vi "eyecat MAX v2-1_JS_160504.vi"() -> ()   [LabVIEW 2014]
doc: "This VI is an upgrade from the WIN 1_v4 that implements the ageing subrutine"
uses:
  Buttons/String output.ctl
  <vilib>/Utility/miscctls.llb/LVRowAndColumnTypeDef.ctl
  Buttons/Numeric control.ctl
  Buttons/String input.ctl
  Buttons/Numeric indicator.ctl
  Controls Win/Control 3.ctl
  <vilib>/Platform/TimedLoop/XDataNode/nitl_modes.ctl
  <vilib>/Platform/TimedLoop/XDataNode/timing_clust.ctl
  <vilib>/Platform/TimedLoop/XDataNode/wakeup.ctl
  <vilib>/Utility/file.llb/Write To Spreadsheet File (string).vi
  <vilib>/Utility/file.llb/Read From Spreadsheet File (string).vi
  <vilib>/Utility/file.llb/Read From Spreadsheet File (DBL).vi
  <vilib>/regexp/Match Regular Expression.xnode
  <vilib>/Platform/TimedLoop/XDataNode/XDataNode.xnode
  <vilib>/Platform/TimedLoop/XDataNode/XDNodeRunTimeDep.lvlib
panel:
  out "Test Loop":dbl
  out "Mexa_One Emissions":dbl[](array[numeric])
  out "Advanced Logging":bool
  out "Full System":bool
  out "MKS":bool
  in  "Alarm":bool
  in  "Analyser":bool
  in  "MFC":bool
  in  "System":bool
  in  "Ageing":bool
  in  "Performance":bool
  in  "Home":bool
  out "NO":dbl[](array[numeric])
  out "CO":dbl[](array[numeric])
  out "Mexa One":bool
  out "Pressure":dbl
  in  "Duration -1":i32
  in  "Demo Sync":i32
  in  "Demo On":bool
  in  "FlowGuide":bool
  in  "Mean(Off)/Interval(On) 2":bool
  in  "Flow Band %":dbl=1.04
  in  "Flow Sync":i32
  out "Emissions":dbl[](array[numeric])
  in  "Temperature Sync":i32
  in  "TempGuide":bool
  in  "Temp Band %":dbl=1.04
  in  "Mean(Off)/Interval(On)":bool
  in  "MKS 5Hz":bool
  out "output cluster":T2
  out "Lambda":dbl[](array[numeric])
  out "MKS HC":dbl
  in  "HC Index":i32
  out "Open/Closed \nLoop":dbl[](array[numeric])
  out "Air Cyc 2":dbl[](array[numeric])
  in  "Cycle size":i32
  out "ExtAnDn":bool
  out "ExtAnUp":bool
  out "HC Cyc 2":dbl[](array[numeric])
  out "SO Valve 2":dbl[](array[numeric])
  out "SO Valve 1":dbl[](array[numeric])
  out "Air Bal":dbl[](array[numeric])
  out "HC Bal":dbl[](array[numeric])
  out "Air Cyc 1":dbl[](array[numeric])
  out "HC Cyc 1":dbl[](array[numeric])
  out "File name":string
  out "Log?":bool
  out "Connected":bool
  out "Furnace temp 2":dbl
  out "Log interval (seconds)":T1
  in  "Flow rate Age":dbl
  in  "Inlet temp Age":dbl
  out "Stopped?":bool
  in  "Stop Cmd":T1
  out "Connected?":bool
  out "Error":dbl
  out "Iteration Duration":i64
  out "Finished Late? [i-1]":bool
  out "Furnace temp 1":dbl
  out "stop 2":bool
  in  "Enum 1":i16=1
  in  "Acknowledge":bool
  out "Test number":u16
  out "Flag1":bool=TRUE
  out "EditPos Subc":T3
  out "Flag 2":bool=TRUE
  in  "Tab Control":T4(tab)
  out "Warm Up":bool
  in  "Leak Test":bool
  in  "Stop Test":bool
  in  "Log Test Data":bool
  in  "Start Test":bool
  in  "Adv Settings":bool
  out "Doors Unlocked":bool
  in  "Temperature Limit (°C)":T1=1200.0 min=0.0 max=1200.0 step=1.0
  in  "File Name":T5="Test"
  in  "File Path":path=path "C:/DATA LOG"
  out "Fail":bool
  out "Pass":bool
  in  "Select Test Type":T6(radio)
  out "Standby":bool
  out "Doors Open":bool
  out "Extractor Fan On":bool
  out "Test In Progress":bool
  out "Cool Down":bool
  out "System Alarm":bool
  in  "Inlet Temperature (°C)":T1=400.0 min=350.0 max=1000.0 step=1.0
  in  "Inlet LAMBDA Rich":T1=0.9 min=0.85 max=0.96 step=0.001
  in  "Inlet LAMBDA Lean":T1=1.2 min=1.02 max=3.0 step=0.001
  in  "Test Stop temperature (°C)":T1=300.0 min=100.0 max=1000.0 step=1.0
  in  "Test Start Temperature (°C)":T1=125.0 min=0.0 max=500.0 step=1.0
  in  "Furnace Ramp Rate (°C/min)":T1=15.0 min=1.0 max=50.0 step=0.1
  in  "NO:CO Ratio":T1=1.1 min=1.0 max=5.0 step=0.1
  in  "Inlet O2 (%)":T1=0.5 min=0.0 max=14.0 step=0.01
  in  "Inlet LAMBDA":T1=1.0 min=0.6 max=3.0 step=0.001
  out "Space Velocity (h-1)":T7
  out "Vol Flow @ STP (l/min)":T7
  in  "Test Flow Rate(g/s)":T1 min=0.0 max=100.0 step=0.01
  out "Sample Volume (litres)":T7
  in  "Number of Samples":T1=1.0 min=1.0 max=6.0 step=1.0
  in  "Sample Diameter (mm)":T1
  out "CO Theory (%)":T7 format="%#_3g"
  out "CO Theory (%)":T7 format="%#_3g"
  out "HC Theory (%)":T7
  in  "Sample Length (mm)":T1 min=0.0 step=0.5
  in  "NO ppm SW":dbl=500.0 caption="NO (ppm)" min=0.0 max=500.0 step=1.0
  in  "NO ppm Loff":T1 caption="NO ppm"
  in  "Delete sCycle":bool
  in  "Load sCycle":bool
  in  "Save sCycle":bool
  in  "Clear subcycle":bool
  in  "Clear Cycle Pattern":bool
  in  "Save Cycle":bool
  in  "Load Cycle":bool
  in  "Delete Cycle":bool
  out "Test Compiled":bool
  in  "Compile Test Button":bool
  in  "Sub-Cycle List":i32(listbox)=1
  in  "Cycle List":i32(listbox)=2
  out "Total Test Duration (hrs)":T8
  in  "Ageing Gas":enum32{"Radio Selection 1", "Radio Selection 2"}(radio)
  in  "Sub-Cycle Pattern":string[][](table) caption="Subcycle pattern"
  in  "Total Number of Cycles":T1=1.0 min=1.0 max=10000.0 step=1.0
  in  "Cycle Pattern":string[][](table)
  in  "Sub-Cycle Name":T5
  in  "Cycle Name":T5
  out "Heat Exchanger Temperatures (°C)":dynamicdata(graph)
  out "Flow Rate (g/s)":dynamicdata(graph)
  out "Sample Temperatures (°C)":dynamicdata(graph)
  out "System Temperatures (°C)":dynamicdata(graph)
  in  "Graph 1 Box":string(combo)="CO"
  in  "Graph 4 Box":string(combo)="NO"
  in  "Graph 3 Box":string(combo)="Air Cycle 1"
  in  "Graph 2 Box":string(combo)="HC Cycle 1"
  out "MFC Graph 4":dynamicdata(graph)
  out "MFC Graph 3":dynamicdata(graph)
  out "MFC Graph 1":dynamicdata(graph)
  out "MFC Graph 2":dynamicdata(graph)
  out "HC Concentration (ppm)":dynamicdata(graph)
  out "Lambda":dynamicdata(graph)
  out "O2/CO Concentration":dynamicdata(graph)
  out "NO Concentration (ppm)":dynamicdata(graph)
  in  "Purge System":bool
  in  "Alarm ack":bool
  in  "Clear log":bool
  out "Table":string[][](table)
  out "Soft Alarm":bool
  out "Hard Alarm":bool
  # "1% = 0.01"
  # "Test Type"
  # "Test Commands"
  # "System Indicators"
  # "Leak Test"
  # "Catalyst Specification"
  # "Lightoff Settings"
  # "Furnace Lightoff Settings"
  # "Sweep Settings"
  # "CO/HC Lightoff Settings"
  # "0.96 < lambda < 0.85"
  # "1.02< lambda < 1.6"
  # "350 < Tinlet < 1000"
  # "NO Lightoff Settings"
  # "Flow Specification"
  # "Cycle Compiled"
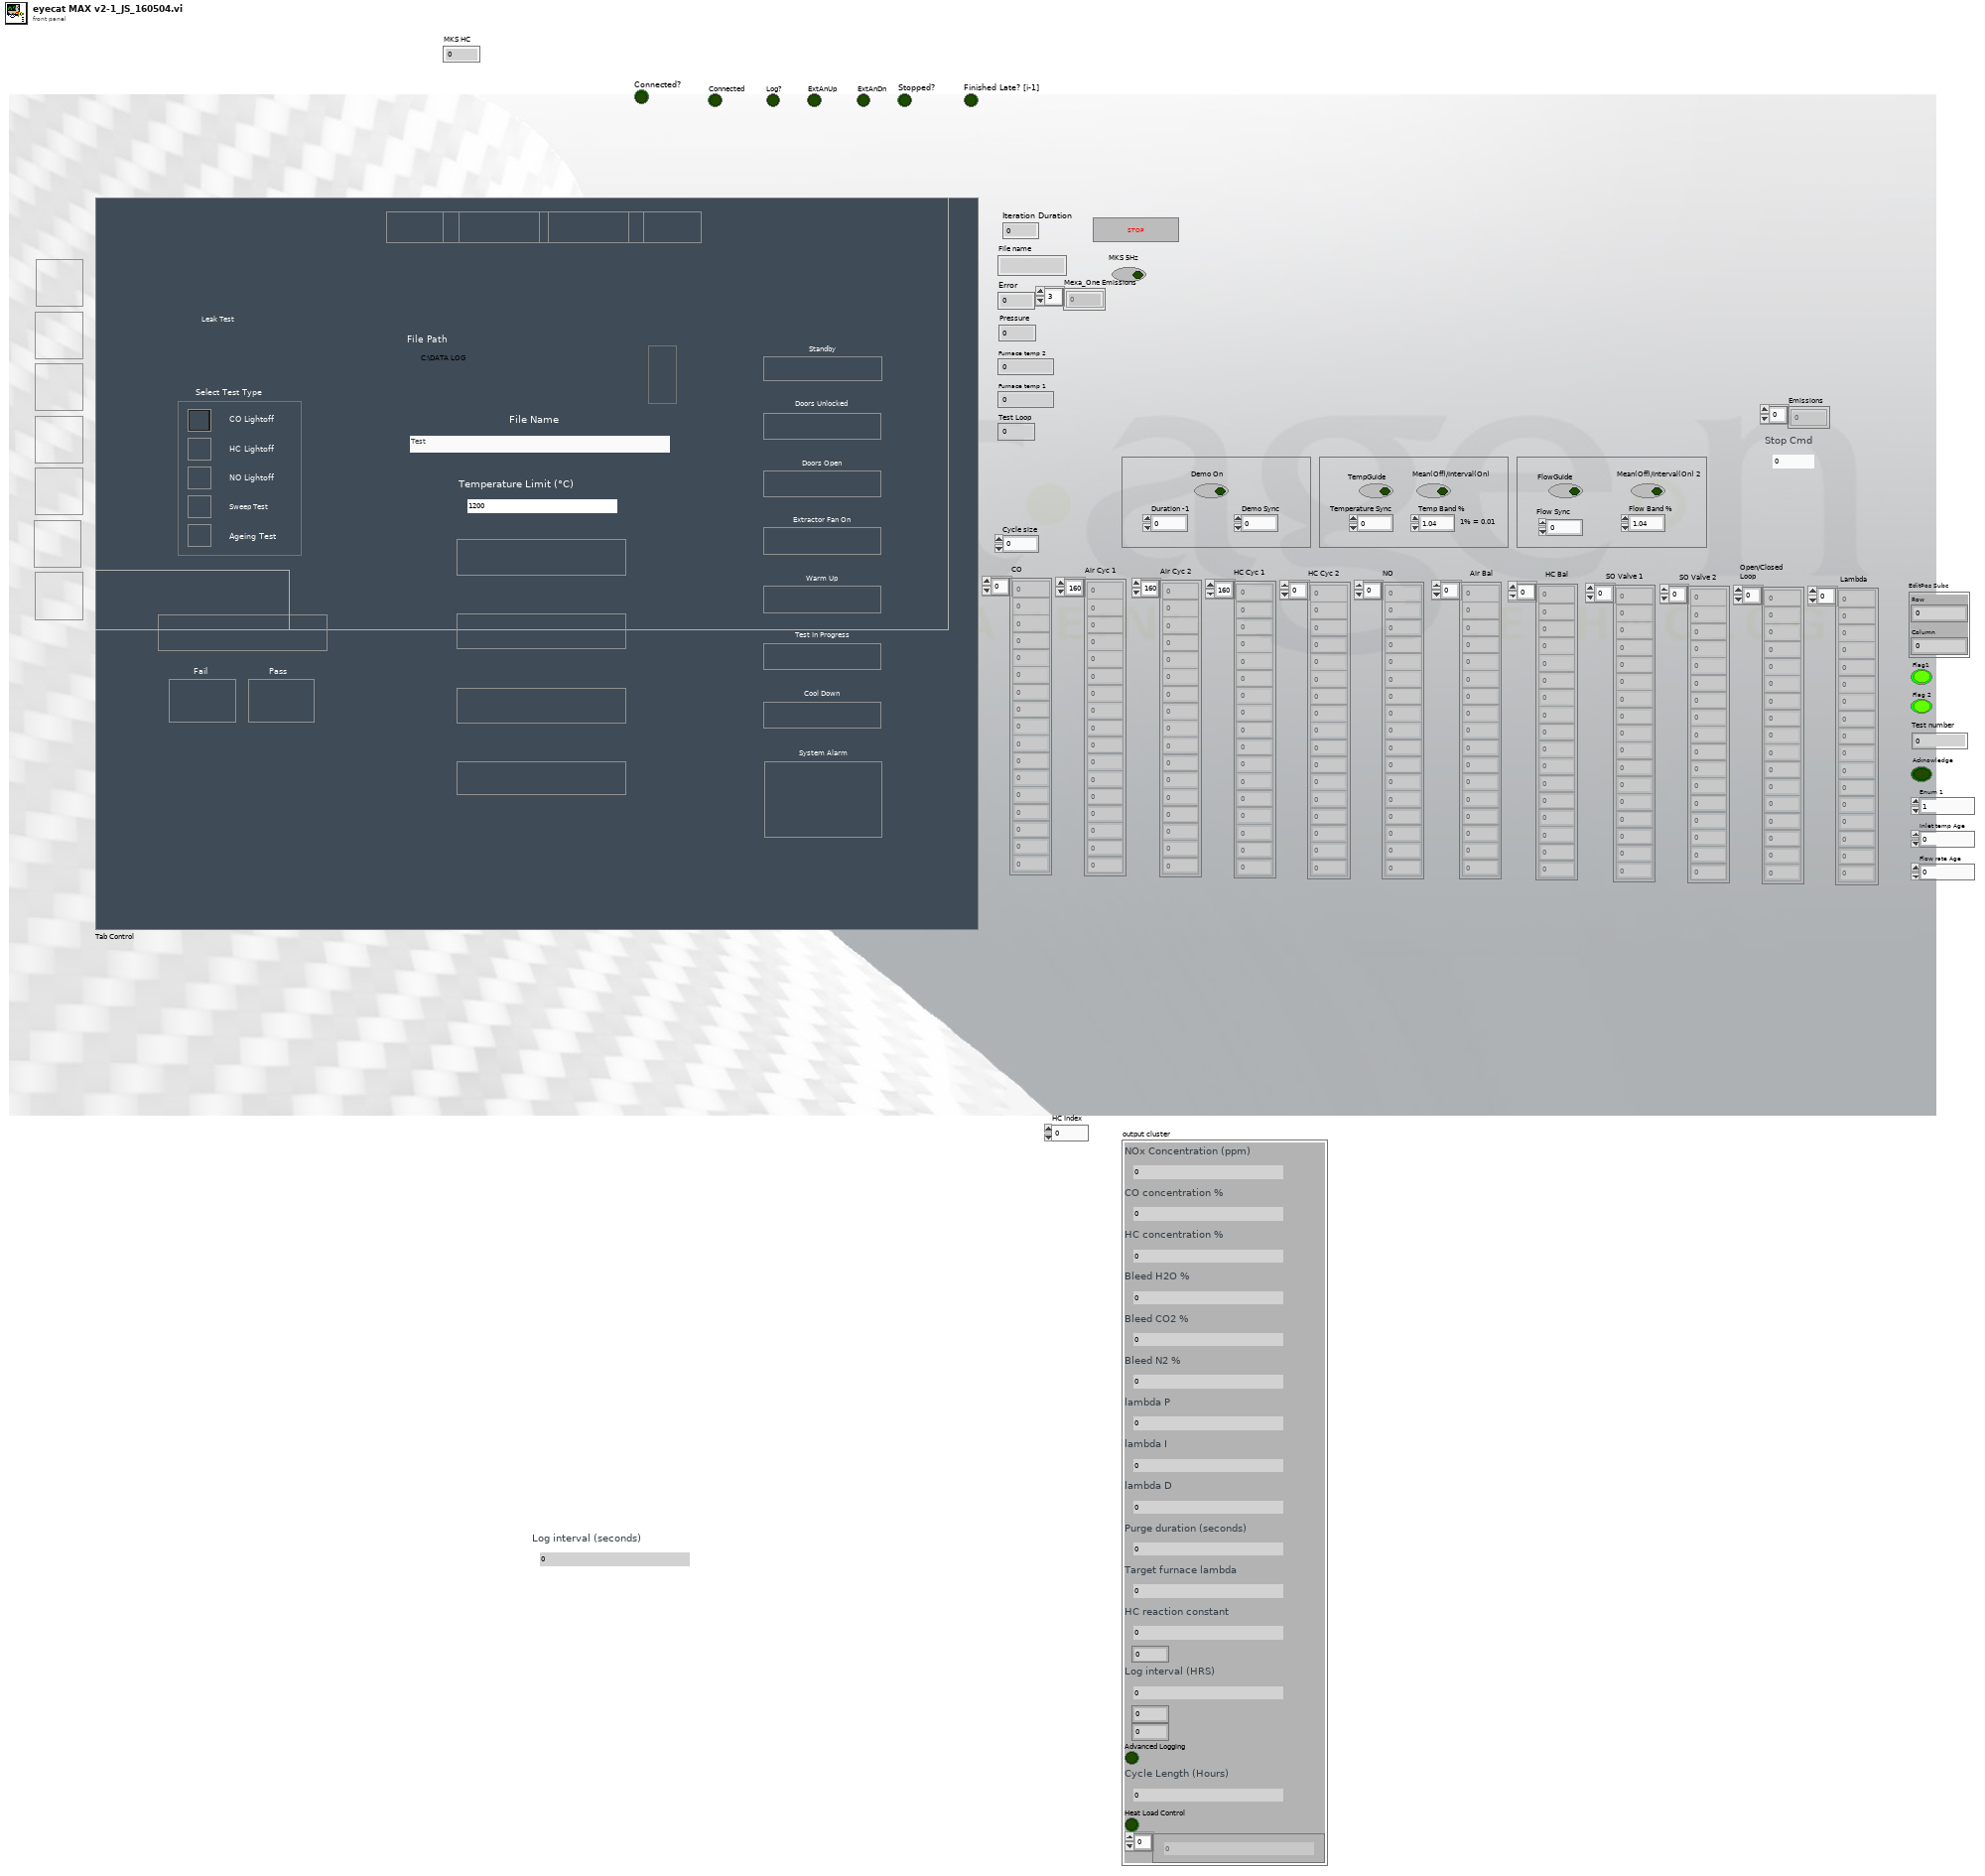
[diagram p1: front panel]
types:
  T1 = typedef "Numeric control.ctl" = dbl
  T2 = cluster{"NOx Concentration (ppm)":T1, "CO concentration %":T1, "HC concentration %":T1, "Bleed H2O %":T1, "Bleed CO2 %":T1, "Bleed N2 %":T1, "lambda P":T1, "lambda I":T1, "lambda D":T1, "Purge duration (seconds)":T1, "Target furnace lambda":T1, "HC reaction constant":T1, i16, "Log interval (HRS)":T1, i16, i16, "Advanced Logging":bool, "Cycle Length (Hours)":T1, "Heat Load Control":bool, T1[]}
  T3 = typedef "LVRowAndColumnTypeDef.ctl" = cluster{"Row":i32, "Column":i32}
  T4 = enum32{"MAIN", "PERFORMANCE TEST SETUP", "AGEING TEST SETUP", "SYSTEM DATA", "MFC", "ANALYSER DATA", "ALARM LOG"}
  T5 = typedef "String input.ctl" = string
  T6 = enum32{"CO Lightoff", "HC Lightoff", "NO Lightoff", "Sweep Test", "Ageing Test"}
  T7 = typedef "Numeric indicator.ctl" = dbl
  T8 = typedef "String output.ctl" = string
  T9 = typedef "XDNodeRunTimeDep.lvlib/nitl_modes.ctl" = enum32{"No Change", "Process missed periods, maintain original phase", "Discard missed periods, maintain original phase", "Process missed periods, ignore original phase", "Discard missed periods, ignore original phase"}
  T10 = typedef "Control 3.ctl" = enum16{"main", "start test", "save subc", "load subc", "delete subc", "clear table 1", "update list 1", "save cycle", "load cycle", "delete cycle", "clear table 2", "update list 2", "calc HC CO", "Total time calc", "update Cycle pattern ", "load cycle name", "convert to num", "load test array", "check scycle name", "check cycle name", "Multigas connect", "Multigas disconnect", "Leak Test"}
  T11 = enum8{"Enabled", "Disabled", "Disabled and Grayed Out"}
  T12 = typedef "XDNodeRunTimeDep.lvlib/timing_clust.ctl" = cluster{"Expected End [f-1]":u64, "Actual End [f-1]":u64, "Finished Late? [f-1]":bool, "Expected End [i-1]":u64, "Actual End [i-1]":u64, "Finished Late? [i-1]":bool, "Expected Start [i]":u64, "Actual Start [i]":u64, "Expected Start [f]":u64, "Actual Start [f]":u64, "Source Name":string, "Structure Name":string, "Period":i64, "Deadline":i64, "Offset":i64, "Start":i64, "Priority":i32, "Timeout":i32, "Mode":T9, "Wakeup Reason":T13, "Error":errorcluster, "Source Type":string, "Secondary Source Type":string, "Global End Time":u64, "Global Start Time":u64, "Frame Duration":u64, "Iteration Duration":u64, "Assigned CPU":i32, "I/O Scan Engine Mode":u32}
  T13 = typedef "XDNodeRunTimeDep.lvlib/wakeup.ctl" = enum32{"Normal", "Aborted", "Asynchronous wakeup", "Timing source error", "Timed loop error", "Timeout"}
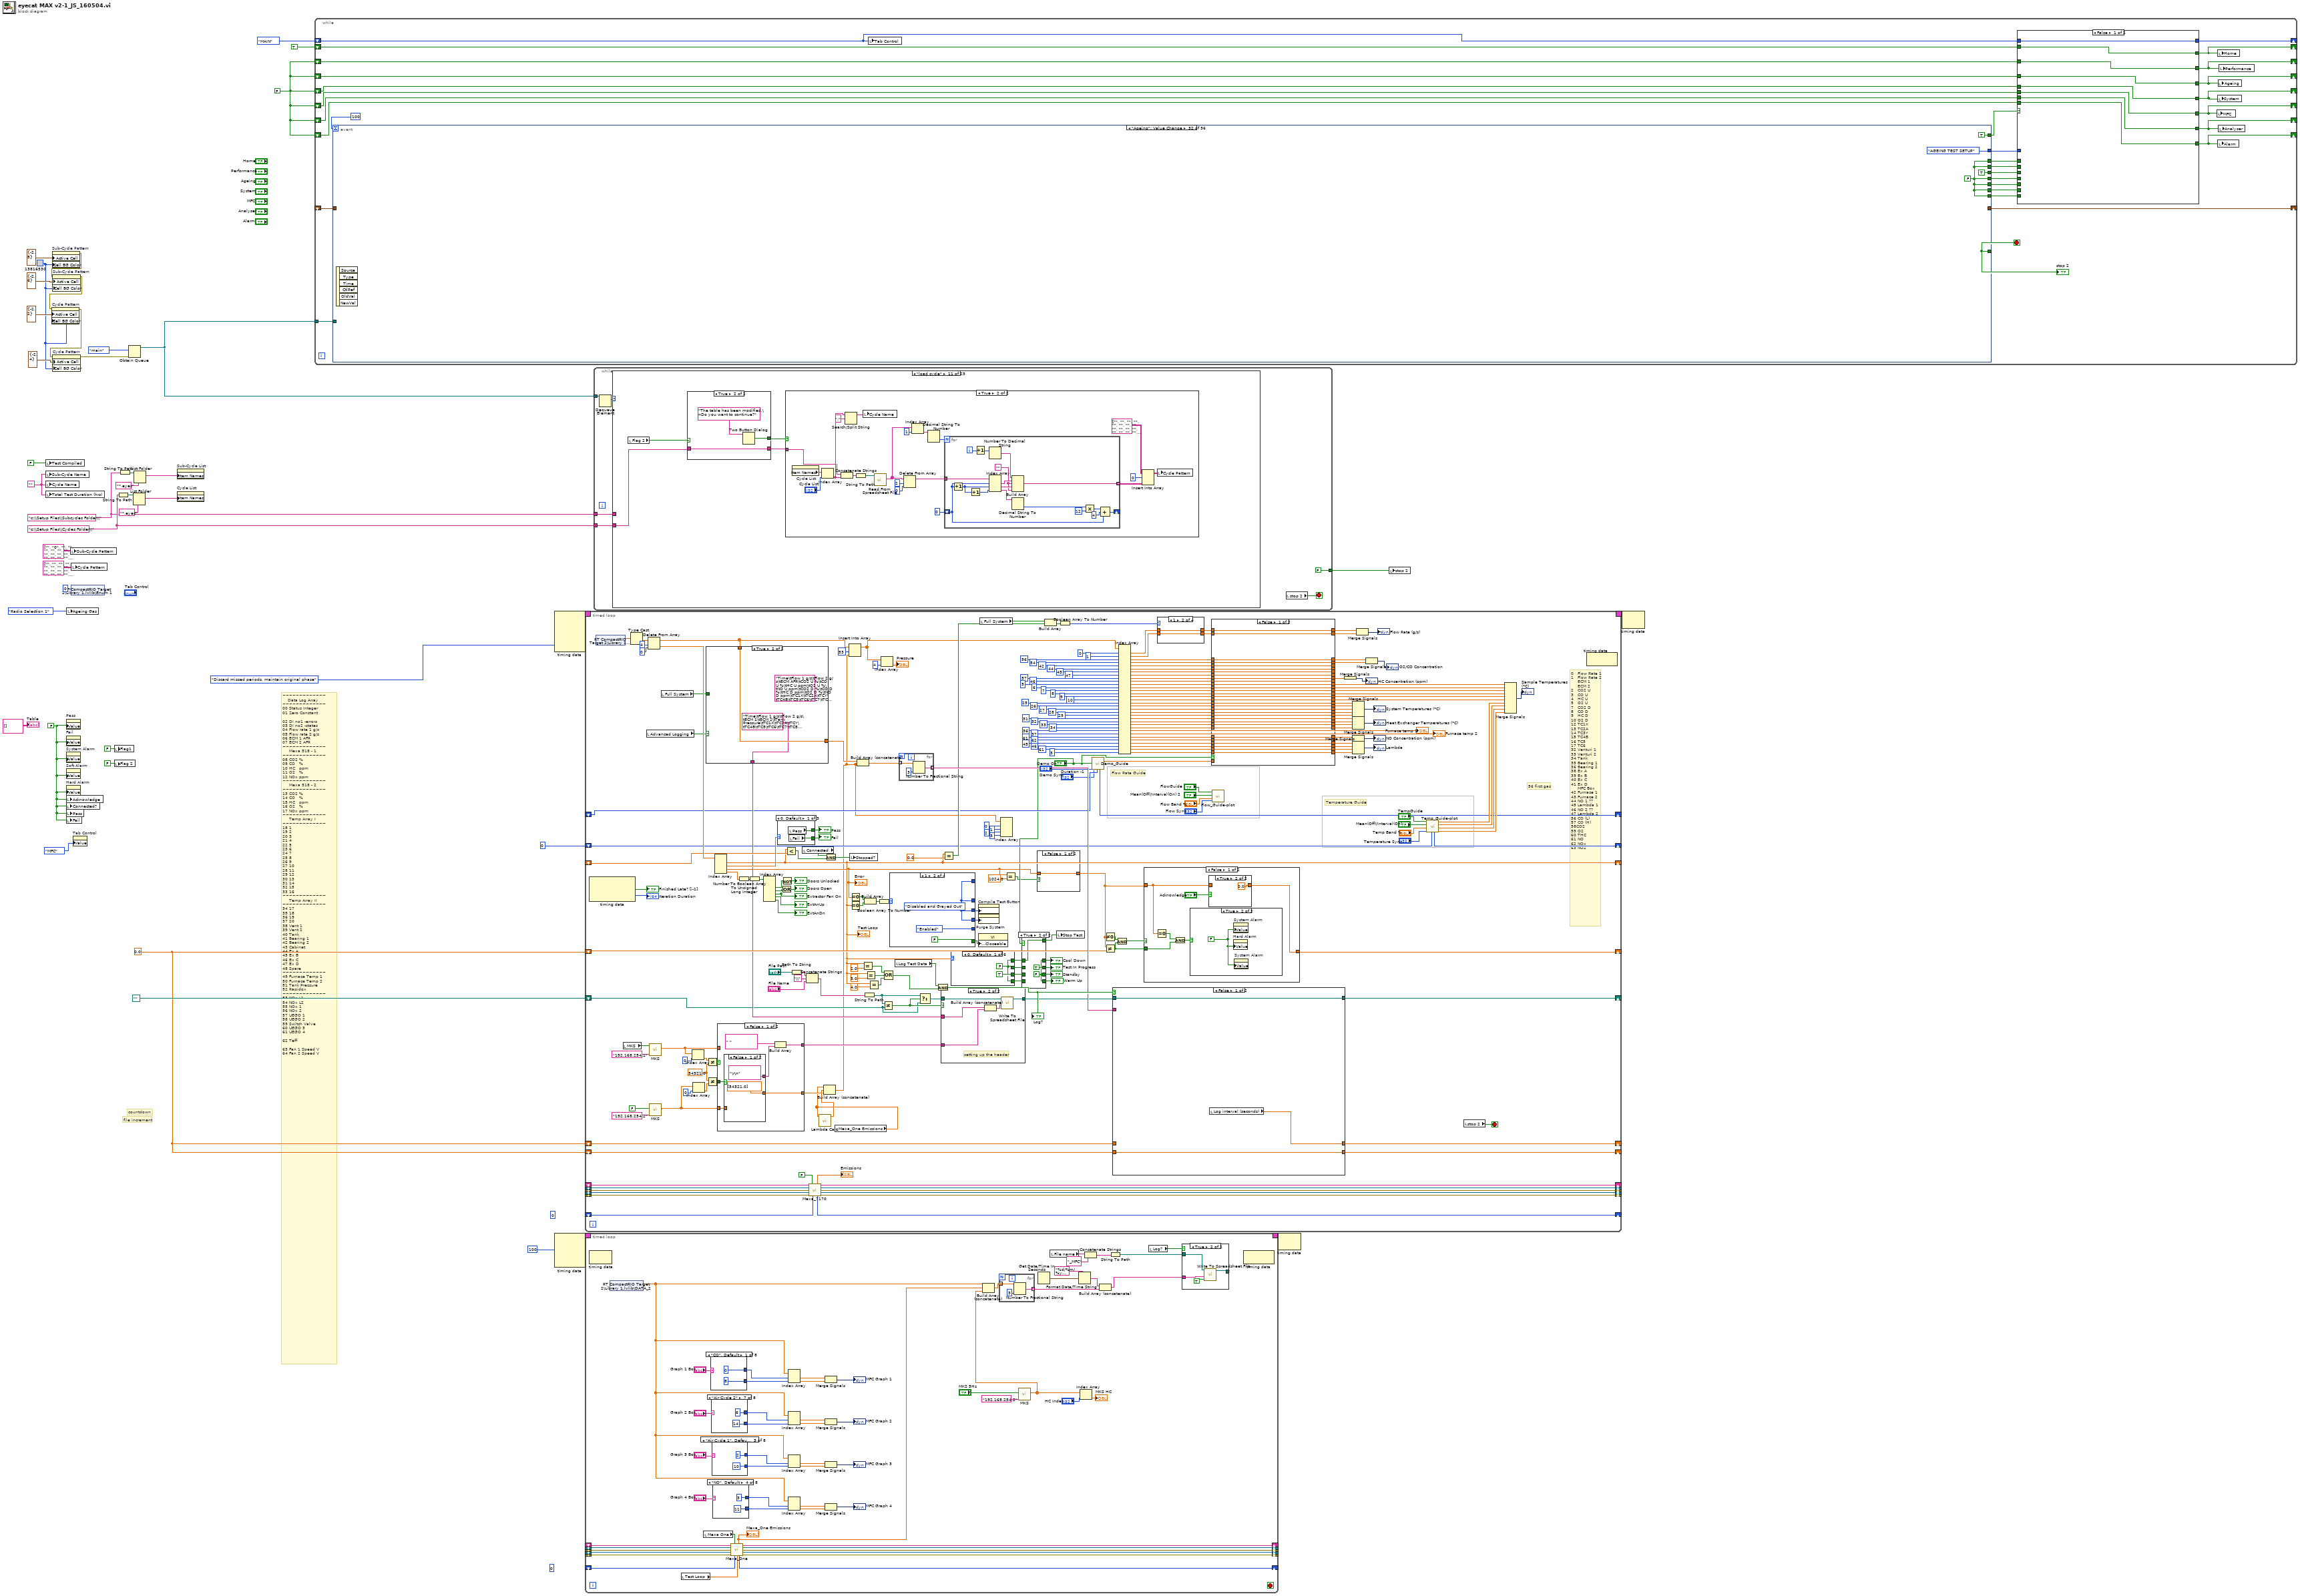
[diagram p0: block diagram]
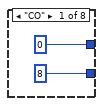
[diagram p2: hidden frame]
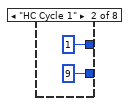
[diagram p3: hidden frame]
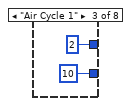
[diagram p4: hidden frame]
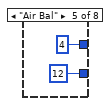
[diagram p5: hidden frame]
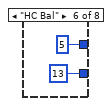
[diagram p6: hidden frame]
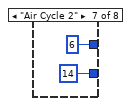
[diagram p7: hidden frame]
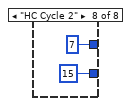
[diagram p8: hidden frame]
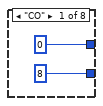
[diagram p9: hidden frame]
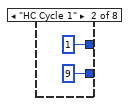
[diagram p10: hidden frame]
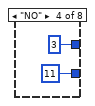
[diagram p11: hidden frame]
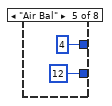
[diagram p12: hidden frame]
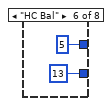
[diagram p13: hidden frame]
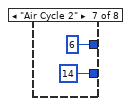
[diagram p14: hidden frame]
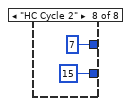
[diagram p15: hidden frame]
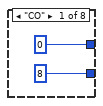
[diagram p16: hidden frame]
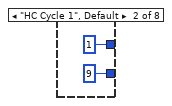
[diagram p17: hidden frame]
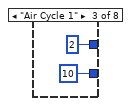
[diagram p18: hidden frame]
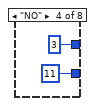
[diagram p19: hidden frame]
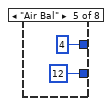
[diagram p20: hidden frame]
diagram:
  (unwired) 0 ("index")
  w2 = FALSE
  (unwired) 0 ("index")
  w10 = FALSE
  w9 = 0.0 ("y")
  w25 = ""
  w28 = "c:\\Setup Files\\Cycles Folder\\"
  w34 = u32 13816530
  w26 = "c:\\Setup Files\\Subcycles Folder\\"
  # "~~~~~~~~~~~~~\n    Data Log Array\n~~~~~~~~~~~~~\n00 Status Integer\n01 Zero Constant\n\n02 DI no1 -errors\n03 DI no2 -states\n04 Flow rate 1 g/s\n05 Flow rate 2 g/s\n06 ECM 1 AFR\n07 ECM 2 AFR\n~~~~~~~~~~~~~\n     Mexa 518 - 1\n~~~~~~~~~~~~~\n08 CO2 %\n09 CO   %\n10 HC   ppm\n11 O2   %\n12 NOx ppm\n~~~~~~~~~~~~~\n     Mexa 518 - 2\n~~~~~~~~~~~~~\n13 CO2 %\n14 CO   %\n15 HC   ppm\n16 O2   %\n17 NOx ppm\n~~~~~~~~~~~~~\n     Temp Array I\n~~~~~~~~~~~~~\n18 1\n19 2 \n20 3\n21 4\n22 5\n23 6\n24 7\n25 8\n26 9\n27 10\n28 11\n29 12\n30 13\n31 14\n32 15\n33 16\n~~~~~~~~~~~~~\n     Temp Array II\n~~~~~~~~~~~~~\n34 17\n35 18\n36 19\n37 20\n38 Vent 1\n39 Vent 2\n40 Tank\n41 Bearing 1\n42 Bearing 2\n43 Cabinet\n44 Ex A\n45 Ex B\n46 Ex C\n47 Ex D\n48 Spare\n~~~~~~~~~~~~~\n49 Furnace Temp 1\n50 Furnace Temp 2\n51 Tank Pressure\n52 Rapidox\n~~~~~~~~~~~~~\n53 NOx L1\n54 NOx L2\n55 NOx 1\n56 NOx 2\n57 UEGO 1\n58 UEGO 2\n59 Switch Valve\n60 UEGO 3\n61 UEGO 4\n\n62 Teff\n\n63 Fan 1 Speed V\n64 Fan 2 Speed V"
  # "file increment"
  # "countdown"
  n1 = local write "Test Compiled"(FALSE ("Cycle Compiled")) -> ()
  n2 = local write "Sub-Cycle Name"(w25) -> ()
  n3 = local write "Cycle Name"(w25) -> ()
  n4 = local write "Total Test Duration (hrs)"(w25) -> ()
  n5 = property on="Sub-Cycle Pattern" class="Tbl (strict)"("Active Cell"=T3 {"Row"=-2, "Column"=5} ("Active Cell:Active Cell"), "Cell BG Color"=w34) -> (error out=w39:errorcluster)  [unwired: 2 in, 1 out]
  n6 = property on="Sub-Cycle Pattern" class="Tbl (strict)"(error in=w39, "Active Cell"=T3 {"Row"=-2, "Column"=6} ("Active Cell:Active Cell"), "Cell BG Color"=w34) -> (error out=w38:errorcluster)  [unwired: 1 in, 1 out]
  n7 = property on="Cycle Pattern" class="Tbl (strict)"(error in=w38, "Active Cell"=T3 {"Row"=-2, "Column"=2} ("Active Cell:Active Cell"), "Cell BG Color"=w34) -> (error out=w36:errorcluster)  [unwired: 1 in, 1 out]
  n8 = property on="Cycle Pattern" class="Tbl (strict)"(error in=w36, "Active Cell"=T3 {"Row"=-2, "Column"=4} ("Active Cell:Active Cell"), "Cell BG Color"=w34) -> (error out=w33:errorcluster)  [unwired: 1 in, 1 out]
  n9 = property on="Pass" class="Bool (strict)"("Value"=w10) -> ()  [unwired: 2 in, 2 out]
  n10 = property on="Fail" class="Bool (strict)"("Value"=w10) -> ()  [unwired: 2 in, 2 out]
  n11 = property on="System Alarm" class="Bool (strict)"("Value"=w10) -> ()  [unwired: 2 in, 2 out]
  n12 = property on="Soft Alarm" class="Bool (strict)"("Value"=w10) -> ()  [unwired: 2 in, 2 out]
  n13 = property on="Hard Alarm" class="Bool (strict)"("Value"=w10) -> ()  [unwired: 2 in, 2 out]
  n14 = local write "Acknowledge"(w10) -> ()
  n15 = local write "Connected?"(w10) -> ()
  n16 = local write "Pass"(w10) -> ()
  n17 = local write "Fail"(w10) -> ()
  n18 = local write "Ageing Gas"(enum32{"Radio Selection 1", "Radio Selection 2"}."Radio Selection 1" ("Ageing Gas")) -> ()
  n19 = local write "Sub-Cycle Pattern"(string[][] [["", "0", "", "", "", "", "", "", "", "", "", "", ""], ["", "", "", "", "", "", "", "", "", "", "", "", ""], ["", "", "", "", "", "", "", "", "", "", "", "", ""], ["", "", "", "", "", "", "", "", "", "", "", "", ""], ["", "", "", "", "", "", "", "", "", "", "", "", ""], ["", "", "", "", "", "", "", "", "", "", "", "", ""], ["", "", "", "", "", "", "", "", "", "", "", "", ""], ["", "", "", "", "", "", "", "", "", "", "", "", ""], ["", "", "", "", "", "", "", "", "", "", "", "", ""], ["", "", "", "", "", "", "", "", "", "", "", "", ""], ["", "", "", "", "", "", "", "", "", "", "", "", ""], ["", "", "", "", "", "", "", "", "", "", "", "", ""], ["", "", "", "", "", "", "", "", "", "", "", "", ""], ["", "", "", "", "", "", "", "", "", "", "", "", ""], ["", "", "", "", "", "", "", "", "", "", "", "", ""], ["", "", "", "", "", "", "", "", "", "", "", "", ""], ["", "", "", "", "", "", "", "", "", "", "", "", ""], ["", "", "", "", "", "", "", "", "", "", "", "", ""], ["", "", "", "", "", "", "", "", "", "", "", "", ""], ["", "", "", "", "", "", "", "", "", "", "", "", ""], ["", "", "", "", "", "", "", "", "", "", "", "", ""], ["", "", "", "", "", "", "", "", "", "", "", "", ""], ["", "", "", "", "", "", "", "", "", "", "", "", ""], ["", "", "", "", "", "", "", "", "", "", "", "", ""], ["", "", "", "", "", "", "", "", "", "", "", "", ""], ["", "", "", "", "", "", "", "", "", "", "", "", ""], ["", "", "", "", "", "", "", "", "", "", "", "", ""], ["", "", "", "", "", "", "", "", "", "", "", "", ""], ["", "", "", "", "", "", "", "", "", "", "", "", ""], ["", "", "", "", "", "", "", "", "", "", "", "", ""], ["", "", "", "", "", "", "", "", "", "", "", "", ""]]) -> ()
  n20 = local write "Cycle Pattern"(string[][] [["", "", "", "", ""], ["", "", "", "", ""], ["", "", "", "", ""], ["", "", "", "", ""], ["", "", "", "", ""], ["", "", "", "", ""], ["", "", "", "", ""], ["", "", "", "", ""], ["", "", "", "", ""], ["", "", "", "", ""], ["", "", "", "", ""], ["", "", "", "", ""], ["", "", "", "", ""], ["", "", "", "", ""], ["", "", "", "", ""], ["", "", "", "", ""], ["", "", "", "", ""], ["", "", "", "", ""], ["", "", "", "", ""], ["", "", "", "", ""], ["", "", "", "", ""], ["", "", "", "", ""], ["", "", "", "", ""], ["", "", "", "", ""], ["", "", "", "", ""], ["", "", "", "", ""], ["", "", "", "", ""], ["", "", "", "", ""], ["", "", "", "", ""], ["", "", "", "", ""], ["", "", "", "", ""]]) -> ()
  n21 = shared-variable "RT CompactRIO Target 2\\Library 1.lvlib\\Enum 1"(u16 0 ("Enum 1")) -> ()  [unwired: 1 in, 1 out]
  n22 = property on="Tab Control" class="TabCtl (strict)"("Value"=T4."MFC" ("Tab Control")) -> ()  [unwired: 2 in, 2 out]
  n23 = local write "Flag1"(FALSE) -> ()
  n24 = local write "Flag 2"(FALSE) -> ()
  n25 = String To Path(string=w28) -> (path=w29:path)
  n26 = String To Path(string=w26) -> (path=w31:path)
  n27 = Obtain Queue(element data type=Control_3."main" ("Enum"), error in (no error)=w33) -> (queue out=w42:refnum<queue>)  [unwired: 3 in, 2 out]
  n28 = List Folder(path=w29, pattern="*.eyec") -> (filenames=w30:string[])  [unwired: 2 in, 3 out]
  n29 = List Folder(path=w31, pattern="*.eyes") -> (filenames=w32:string[])  [unwired: 2 in, 3 out]
  n30 = property on="Sub-Cycle List" class="LstBox (strict)"("Item Names"=w32) -> ()  [unwired: 2 in, 2 out]
  n31 = property on="Cycle List" class="LstBox (strict)"("Item Names"=w30) -> ()  [unwired: 2 in, 2 out]
  n32 = while {
    tunnel: w42 -> [w73]
    shift-right: [w71] -> _
    shift-left: _ -> [w70]
    shift-right: [w68] -> _
    shift-left: T4."MAIN" ("Tab Control") -> [w67]
    shift-right: [w56] -> _
    shift-left: w2 -> [w49]
    shift-right: [w57] -> _
    shift-left: TRUE -> [w50]
    shift-right: [w55] -> _
    shift-left: w2 -> [w44]
    shift-right: [w54] -> _
    shift-left: w2 -> [w45]
    shift-right: [w53] -> _
    shift-left: w2 -> [w46]
    shift-right: [w52] -> _
    shift-left: w2 -> [w47]
    shift-right: [w51] -> _
    shift-left: w2 -> [w48]
    stop <- w69 stop-if-true
    n33 = event shown="[31] \"Ageing\": Value Change" {
      selector: _ -> [_ _ _ _ _ _ _ _ _ _ _ _ _ _ _ _ _ _ _ _ _ _ _ _ _ _ _ _ _ _ _ _ _ _ _ _]
      dyn-events: _ -> [_ _ _ _ _ _ _ _ _ _ _ _ _ _ _ _ _ _ _ _ _ _ _ _ _ _ _ _ _ _ _ _ _ _ _ _]
      timeout: 100 -> [_ _ _ _ _ _ _ _ _ _ _ _ _ _ _ _ _ _ _ _ _ _ _ _ _ _ _ _ _ _ _ _ _ _ _ _]
      tunnel: w73 -> [w92 w94 _ w103 w111 w118 w125 w136 w140 w151 w156 w159 w164 w186 w194 w195 _ _ _ _ w239 w250 _ w342 w366 _ w380 _ _ _ _ _ _ _ _ _]
      tunnel: [w90 w93 _ w104 w110 w117 w124 w135 w138 w146 w153 w158 w162 w183 _ _ _ _ _ _ _ _ _ _ _ _ _ _ _ _ _ _ _ _ _ _] -> w71
      tunnel: w70 -> [w90 w93 _ w104 w110 w117 w123 w135 w138 w146 w153 w158 w162 w183 _ _ _ _ _ _ _ _ _ _ _ _ _ _ _ _ _ _ _ _ _ _]
      tunnel: [_ _ w96 _ _ _ _ _ _ _ _ _ _ _ _ _ _ _ _ _ _ _ _ _ _ _ _ _ _ _ _ _ _ _ _ _] -> w69
      tunnel: [_ _ _ _ _ _ _ _ _ _ _ _ _ _ _ _ _ _ _ _ _ _ _ _ _ _ _ _ _ TRUE TRUE TRUE TRUE TRUE TRUE TRUE] -> w66
      tunnel: [_ _ _ _ _ _ _ _ _ _ _ _ _ _ _ _ _ _ _ _ _ _ _ _ _ _ _ _ _ T4."MAIN" ("Tab Control") T4."PERFORMANCE TEST SETUP" ("Tab Control") T4."AGEING TEST SETUP" ("Tab Control") T4."SYSTEM DATA" ("Tab Control") T4."MFC" ("Tab Control") T4."ANALYSER DATA" ("Tab Control") T4."ALARM LOG" ("Tab Control")] -> w65
      tunnel: [_ _ _ _ _ _ _ _ _ _ _ _ _ _ _ _ _ _ _ _ _ _ _ _ _ _ _ _ _ TRUE w391 w395 w399 w403 w408 w411] -> w64
      tunnel: [_ _ _ _ _ _ _ _ _ _ _ _ _ _ _ _ _ _ _ _ _ _ _ _ _ _ _ _ _ w388 TRUE w395 w399 w403 w408 w411] -> w63
      tunnel: [_ _ _ _ _ _ _ _ _ _ _ _ _ _ _ _ _ _ _ _ _ _ _ _ _ _ _ _ _ w388 w391 TRUE w399 w403 w408 w411] -> w62
      tunnel: [_ _ _ _ _ _ _ _ _ _ _ _ _ _ _ _ _ _ _ _ _ _ _ _ _ _ _ _ _ w388 w391 w395 TRUE w403 w408 w411] -> w61
      tunnel: [_ _ _ _ _ _ _ _ _ _ _ _ _ _ _ _ _ _ _ _ _ _ _ _ _ _ _ _ _ w388 w391 w395 w399 TRUE w408 w411] -> w60
      tunnel: [_ _ _ _ _ _ _ _ _ _ _ _ _ _ _ _ _ _ _ _ _ _ _ _ _ _ _ _ _ w388 w391 w395 w399 w403 TRUE w411] -> w59
      tunnel: [_ _ _ _ _ _ _ _ _ _ _ _ _ _ _ _ _ _ _ _ _ _ _ _ _ _ _ _ _ w388 w391 w395 w399 w403 w408 TRUE] -> w58
      event Timeout {
        n34 = event-data() -> ()  [unwired: 1 in, 2 out]
        n35 = Enqueue Element(queue=w92, element=Control_3."main" ("Enum")) -> ()  [unwired: 2 in, 3 out]
      }
      event "Clear subcycle": Value Change {
        n36 = event-data() -> ()  [unwired: 1 in, 5 out]
        n37 = Enqueue Element(queue=w94, element=Control_3."clear table 1" ("Enum")) -> ()  [unwired: 2 in, 3 out]
      }
      event Panel Close? {
        n38 = event-data() -> ()  [unwired: 1 in, 3 out]
        n39 = Two Button Dialog(message="This command will close Eyecat!\nDo you wish to continue?", 1:"No" ("F button name (\"Cancel\")"), 2:"Yes" ("T button name (\"OK\")")) -> (T button?=w96:bool)
        n40 = Not(x=w96) -> (.not. x?=w97:bool)
        n41 = event-data("Discard?"=w97) -> ()  [unwired: 1 in, 1 out]
      }
      event "Save sCycle": Value Change {
        n42 = event-data() -> ()  [unwired: 1 in, 5 out]
        n43 = local read "Sub-Cycle Pattern"() -> (w101:string[][])
        n44 = call "Time column check.vi"("Array"=w101) -> ("Mistake?"=w102:bool)  [unwired: 10 in]
        n45 = case shown="False" w102 {
          tunnel: w103 -> [w105 _]
          frame False {
            n46 = Enqueue Element(queue=w105, element=Control_3."save subc") -> (queue out=w107:refnum<queue>)  [unwired: 2 in, 2 out]
            n47 = Enqueue Element(queue=w107, element=Control_3."update list 1") -> ()  [unwired: 2 in, 3 out]
          }
          frame True {
            n48 = One Button Dialog(message="The time sequence is incorrect!\nReview and save again!") -> ()  [unwired: 1 in, 1 out]
          }
        }
      }
      event "Load sCycle": Value Change {
        n49 = event-data() -> ()  [unwired: 1 in, 5 out]
        n50 = Enqueue Element(queue=w111, element=Control_3."load subc") -> ()  [unwired: 2 in, 3 out]
      }
      event "Delete sCycle": Value Change {
        n51 = event-data() -> ()  [unwired: 1 in, 5 out]
        n52 = Enqueue Element(queue=w118, element=Control_3."delete subc") -> (queue out=w120:refnum<queue>)  [unwired: 2 in, 2 out]
        n53 = Enqueue Element(queue=w120, element=Control_3."update list 1") -> (queue out=w116:refnum<queue>)  [unwired: 2 in, 2 out]
        n54 = Enqueue Element(queue=w116, element=Control_3."update Cycle pattern ") -> (queue out=w113:refnum<queue>)  [unwired: 2 in, 2 out]
        n55 = Enqueue Element(queue=w113, element=Control_3."Total time calc") -> ()  [unwired: 2 in, 3 out]
      }
      event "Sub-Cycle Pattern": Mouse Down; "Sub-Cycle Pattern": Value Change {
        n56 = event-data() -> ()  [unwired: 1 in, 3 out]
        n57 = property on="Sub-Cycle Pattern" class="Tbl (strict)"() -> ("EditPos"=w124:T3)  [unwired: 2 in, 2 out]
        n58 = Unbundle By Name(w124) -> ("Row"=w126:i32)  [unwired: 1 out]
        n59 = Less?(x=w126, y=30) -> (x < y?=w128:bool)
        n60 = case shown="True" w128 {
          tunnel: w125 -> [_ w133]
          frame False {
            n61 = One Button Dialog(message="This table is limited to 30 entries!") -> ()  [unwired: 1 in, 1 out]
          }
          frame True {
            n62 = Enqueue Element(queue=w133, element=Control_3."convert to num") -> (queue out=w132:refnum<queue>)  [unwired: 2 in, 2 out]
            n63 = Enqueue Element(queue=w132, element=Control_3."calc HC CO") -> ()  [unwired: 2 in, 3 out]
          }
        }
        "EditPos Subc" <- w123
        "Flag1" <- TRUE
      }
      event "Clear Cycle Pattern": Value Change {
        n64 = event-data() -> ()  [unwired: 1 in, 5 out]
        n65 = Enqueue Element(queue=w136, element=Control_3."clear table 2" ("Enum")) -> ()  [unwired: 2 in, 3 out]
        n66 = local write "Test Compiled"(FALSE ("Test Compiled")) -> ()
      }
      event "Save Cycle": Value Change {
        n67 = event-data() -> ()  [unwired: 1 in, 5 out]
        n68 = Enqueue Element(queue=w140, element=Control_3."update Cycle pattern ") -> (queue out=w139:refnum<queue>)  [unwired: 2 in, 2 out]
        n69 = Enqueue Element(queue=w139, element=Control_3."save cycle") -> (queue out=w143:refnum<queue>)  [unwired: 2 in, 2 out]
        n70 = Enqueue Element(queue=w143, element=Control_3."update list 2") -> ()  [unwired: 2 in, 3 out]
      }
      event "Load Cycle": Value Change {
        n71 = event-data() -> ()  [unwired: 1 in, 5 out]
        n72 = Enqueue Element(queue=w151, element=Control_3."load cycle") -> (queue out=w149:refnum<queue>)  [unwired: 2 in, 2 out]
        n73 = Enqueue Element(queue=w149, element=Control_3."update Cycle pattern ") -> (queue out=w148:refnum<queue>)  [unwired: 2 in, 2 out]
        n74 = local write "Test Compiled"(FALSE ("Test Compiled")) -> ()
        n75 = Enqueue Element(queue=w148, element=Control_3."Total time calc") -> ()  [unwired: 2 in, 3 out]
      }
      event "Delete Cycle": Value Change {
        n76 = event-data() -> ()  [unwired: 1 in, 5 out]
        n77 = Enqueue Element(queue=w156, element=Control_3."delete cycle") -> (queue out=w155:refnum<queue>)  [unwired: 2 in, 2 out]
        n78 = Enqueue Element(queue=w155, element=Control_3."update list 2") -> ()  [unwired: 2 in, 3 out]
      }
      event Value Change {
        n79 = event-data() -> ()  [unwired: 1 in, 5 out]
        n80 = Enqueue Element(queue=w159, element=Control_3."Total time calc") -> ()  [unwired: 2 in, 3 out]
      }
      event "Cycle Pattern": Mouse Up; "Cycle Pattern": Value Change {
        n81 = event-data() -> ()  [unwired: 1 in, 3 out]
        n82 = property on="Cycle Pattern" class="Tbl (strict)"() -> ("EditPos"=w166:T3)  [unwired: 2 in, 2 out]
        n83 = Unbundle By Name(w166) -> ("Row"=w163:i32, "Column"=w168:i32)
        n84 = Less?(x=w163, y=30) -> (x < y?=w167:bool)
        n85 = case shown="True" w167 {
          tunnel: w168 -> [_ w170]
          tunnel: w164 -> [_ w173]
          frame False {
            n86 = One Button Dialog(message="This table is limited to 30 entries!") -> ()  [unwired: 1 in, 1 out]
          }
          frame True {
            n87 = Equal?(x=w170, y=1) -> (x = y?=w174:bool)
            n88 = case shown="True" w174 {
              tunnel: w173 -> [w177 w180]
              tunnel: [w176 w179] -> w172
              frame False {
                n89 = Enqueue Element(queue=w177, element=Control_3."update Cycle pattern ") -> (queue out=w176:refnum<queue>)  [unwired: 2 in, 2 out]
              }
              frame True {
                n90 = Enqueue Element(queue=w180, element=Control_3."load cycle name") -> (queue out=w179:refnum<queue>)  [unwired: 2 in, 2 out]
              }
            }
            n91 = Enqueue Element(queue=w172, element=Control_3."Total time calc") -> ()  [unwired: 2 in, 3 out]
          }
        }
        "Flag 2" <- TRUE
      }
      event "Compile Test Button": Value Change {
        n92 = event-data() -> ()  [unwired: 1 in, 5 out]
        n93 = local read "Flag 2"() -> (w182:bool)
        n94 = case shown="True" w182 {
          tunnel: w186 -> [w187 w191]
          tunnel: [w187 w188] -> w184
          frame False {
          }
          frame True {
            n95 = Enqueue Element(queue=w191, element=Control_3."save cycle") -> (queue out=w189:refnum<queue>)  [unwired: 2 in, 2 out]
            n96 = Enqueue Element(queue=w189, element=Control_3."update list 2") -> (queue out=w188:refnum<queue>)  [unwired: 2 in, 2 out]
          }
        }
        n97 = Enqueue Element(queue=w184, element=Control_3."load test array") -> ()  [unwired: 2 in, 3 out]
      }
      event Value Change {
        n98 = event-data() -> ()  [unwired: 1 in, 5 out]
        n99 = Enqueue Element(queue=w194, element=Control_3."check scycle name") -> ()  [unwired: 2 in, 3 out]
      }
      event Value Change {
        n100 = event-data() -> ()  [unwired: 1 in, 5 out]
        n101 = Enqueue Element(queue=w195, element=Control_3."check cycle name") -> ()  [unwired: 2 in, 3 out]
      }
      event Value Change {
        n102 = event-data() -> ()  [unwired: 1 in, 5 out]
        n103 = Square(x="Sample Diameter (mm)") -> (x^2=w204:T1)
        n104 = Compound Arithmetic op=MULTIPLY(w204, "Sample Length (mm)", "Number of Samples", 3.141592653589793) -> (w203:T1)
        n105 = Divide(x=w203, y=4000000.0) -> (x/y=→"Sample Volume (litres)":T1)
      }
      event Value Change {
        # "O2Eq"
        n106 = event-data() -> ()  [unwired: 1 in, 5 out]
        n107 = local write "Inlet LAMBDA"("Inlet LAMBDA") -> ()
        n108 = local write "Inlet O2 (%)"("Inlet O2 (%)") -> ()
        n109 = Decrement(x="Inlet LAMBDA") -> (x-1=w219:T1)
        n110 = Multiply(x=4.76, y="Inlet LAMBDA") -> (x*y=w215:T1)
        n111 = Multiply(x=w219, y=100.0) -> (x*y=w217:T1)
        n112 = Add(x=0.33, y=w215) -> (x+y=w213:T1)
        n113 = Divide(x=w217, y=w213) -> (x/y=w212:T1)
        n114 = Subtract(x="Inlet O2 (%)", y=w212) -> (x-y=w210:T1)
        n115 = Multiply(x=w210, y=2.0) -> (x*y=→"CO Theory (%)":T1)
        n116 = Divide(x=w210, y=4.5) -> (x/y=→"HC Theory (%)":T1)
      }
      event Value Change {
        n117 = event-data() -> ()  [unwired: 1 in, 5 out]
        n118 = local write "NO ppm Loff"("NO ppm Loff") -> ()
        n119 = local write "NO:CO Ratio"("NO:CO Ratio") -> ()
        n120 = Divide(x="NO ppm Loff", y=T1 10000.0) -> (x/y=w222:T1)
        n121 = Multiply(x="NO:CO Ratio", y=w222) -> (x*y=→"CO Theory (%)":T1)
      }
      event Value Change {
        n122 = event-data() -> ()  [unwired: 1 in, 5 out]
        n123 = local read "Sample Volume (litres)"() -> (w227:T7)
        n124 = Equal?(x=w227, y=0.0) -> (x = y?=w226:bool)
        n125 = case shown="False" w226 {
          tunnel: w227 -> [w232 _]
          tunnel: "Test Flow Rate(g/s)" -> [w229 _]
          frame False {
            w234 = 60.0 ("y")
            n126 = Multiply(x=w229, y=w234) -> (x*y=w236:T1)
            n127 = Divide(x=w236, y=1.2) -> (x/y=w231:T1)
            "Vol Flow @ STP (l/min)" <- w231
            n128 = Multiply(x=w231, y=w234) -> (x*y=w233:T1)
            n129 = Divide(x=w233, y=w232) -> (x/y=→"Space Velocity (h-1)":T1)
          }
          frame True {
            n130 = One Button Dialog(message="Review sample specification first!") -> ()  [unwired: 1 in, 1 out]
          }
        }
      }
      event "Leak Test": Value Change {
        n131 = event-data() -> ()  [unwired: 1 in, 5 out]
        n132 = flat-sequence {
          tunnel: w239 -> [w242]
          tunnel: [w242] -> w238
          tunnel: w238 -> [w247]
          frame #0 {
            n133 = local write "Test number"(u16 5) -> ()
            n134 = local write "Enum 1"(u16 3 ("Test number")) -> ()
          }
          frame #1 {
            n135 = Enqueue Element(queue=w247, element=Control_3."main" ("Enum")) -> (queue out=w245:refnum<queue>)  [unwired: 2 in, 2 out]
            n136 = Enqueue Element(queue=w245, element=Control_3."start test" ("Enum")) -> (queue out=w244:refnum<queue>)  [unwired: 2 in, 2 out]
            n137 = Enqueue Element(queue=w244, element=Control_3."Leak Test" ("Enum")) -> ()  [unwired: 2 in, 3 out]
          }
        }
      }
      event "Start Test": Value Change {
        n138 = event-data() -> ()  [unwired: 1 in, 6 out]
        n139 = case shown="True" "Start Test" {
          tunnel: w250 -> [_ w259]
          frame False {
          }
          frame True {
            n140 = local read "Log Test Data"() -> (w251:bool)
            n141 = Boolean To (0,1)(Boolean=w251) -> (0, 1=w258:i16)
            n142 = Equal To 0?(x=w258) -> (x = 0?=w257:bool)
            n143 = case shown="True" w257 {
              tunnel: [TRUE ("T button?") w261] -> w252
              frame False {
              }
              frame True {
                # "Log Data Check"
                n144 = Two Button Dialog(message="You are not currently logging data!\nDo you wish to continue?", 1:"No" ("T button name (\"OK\")"), 2:"Yes" ("T button name (\"OK\")")) -> (T button?=w261:bool)
              }
            }
            n145 = Equal?(x=2.0, y=2.0) -> (x = y?=w253:bool)
            n146 = And(x=w253, y=w252) -> (x .and. y?=w254:bool)
            n147 = case shown="True" w254 {
              frame False {
              }
              frame True {
                n148 = flat-sequence {
                  tunnel: "Cycle size" -> [w288]
                  tunnel: [w288] -> w277
                  tunnel: [w291] -> w286
                  tunnel: w277 -> [w291]
                  tunnel: w286 -> [w294]
                  tunnel: [w294] -> w285
                  tunnel: w285 -> [w297]
                  tunnel: [w297] -> w284
                  tunnel: w284 -> [w300]
                  tunnel: [w300] -> w276
                  tunnel: w276 -> [w303]
                  tunnel: [w303] -> w275
                  tunnel: [w306] -> w287
                  tunnel: w275 -> [w306]
                  tunnel: [w309] -> w283
                  tunnel: w287 -> [w309]
                  tunnel: w283 -> [w312]
                  tunnel: [w312] -> w281
                  tunnel: w281 -> [w315]
                  tunnel: [w315] -> w280
                  tunnel: w280 -> [w318]
                  tunnel: [w318] -> w279
                  tunnel: w279 -> [w324]
                  tunnel: [w324] -> w278
                  tunnel: w278 -> [w335]
                  frame #0 {
                    n149 = call-poly <vilib>:"Read From Spreadsheet File.vi"() -> ("all rows"=w289:dbl[][])  [unwired: 7 in, 4 out]
                    n150 = Reshape Array(w289, w288) -> (→"CO":dbl[])
                  }
                  frame #1 {
                    n151 = call-poly <vilib>:"Read From Spreadsheet File.vi"() -> ("all rows"=w293:dbl[][])  [unwired: 7 in, 4 out]
                    n152 = Reshape Array(w293, w291) -> (→"Air Cyc 1":dbl[])
                  }
                  frame #2 {
                    n153 = call-poly <vilib>:"Read From Spreadsheet File.vi"() -> ("all rows"=w295:dbl[][])  [unwired: 7 in, 4 out]
                    n154 = Reshape Array(w295, w294) -> (→"Air Cyc 2":dbl[])
                  }
                  frame #3 {
                    n155 = call-poly <vilib>:"Read From Spreadsheet File.vi"() -> ("all rows"=w299:dbl[][])  [unwired: 7 in, 4 out]
                    n156 = Reshape Array(w299, w297) -> (→"HC Cyc 1":dbl[])
                  }
                  frame #4 {
                    n157 = call-poly <vilib>:"Read From Spreadsheet File.vi"() -> ("all rows"=w302:dbl[][])  [unwired: 7 in, 4 out]
                    n158 = Reshape Array(w302, w300) -> (→"HC Cyc 2":dbl[])
                  }
                  frame #5 {
                    n159 = call-poly <vilib>:"Read From Spreadsheet File.vi"() -> ("all rows"=w304:dbl[][])  [unwired: 7 in, 4 out]
                    n160 = Reshape Array(w304, w303) -> (→"NO":dbl[])
                  }
                  frame #6 {
                    n161 = call-poly <vilib>:"Read From Spreadsheet File.vi"() -> ("all rows"=w307:dbl[][])  [unwired: 7 in, 4 out]
                    n162 = Reshape Array(w307, w306) -> (→"Air Bal":dbl[])
                  }
                  frame #7 {
                    n163 = call-poly <vilib>:"Read From Spreadsheet File.vi"() -> ("all rows"=w311:dbl[][])  [unwired: 7 in, 4 out]
                    n164 = Reshape Array(w311, w309) -> (→"HC Bal":dbl[])
                  }
                  frame #8 {
                    n165 = call-poly <vilib>:"Read From Spreadsheet File.vi"() -> ("all rows"=w313:dbl[][])  [unwired: 7 in, 4 out]
                    n166 = Reshape Array(w313, w312) -> (→"SO Valve 1":dbl[])
                  }
                  frame #9 {
                    n167 = call-poly <vilib>:"Read From Spreadsheet File.vi"() -> ("all rows"=w316:dbl[][])  [unwired: 7 in, 4 out]
                    n168 = Reshape Array(w316, w315) -> (→"SO Valve 2":dbl[])
                  }
                  frame #10 {
                    n169 = call-poly <vilib>:"Read From Spreadsheet File.vi"() -> ("all rows"=w320:dbl[][])  [unwired: 7 in, 4 out]
                    n170 = Reshape Array(w320, w318) -> (→"Open/Closed \nLoop":dbl[])
                  }
                  frame #11 {
                    n171 = local read "Open/Closed \nLoop"() -> (w325:dbl[])
                    n172 = local read "SO Valve 1"() -> (w327:dbl[])
                    n173 = local read "SO Valve 2"() -> (w326:dbl[])
                    n174 = local read "HC Cyc 2"() -> (w330:dbl[])
                    n175 = local read "HC Cyc 1"() -> (w329:dbl[])
                    n176 = local read "Air Cyc 1"() -> (w323:dbl[])
                    n177 = local read "Air Cyc 2"() -> (w328:dbl[])
                    n178 = local read "HC Bal"() -> (w332:dbl[])
                    n179 = local read "Air Bal"() -> (w331:dbl[])
                    n180 = local read "NO"() -> (w321:dbl[])
                    n181 = local read "CO"() -> (w322:dbl[])
                    n182 = Build Array (concatenate)(w324, w322, w323, w328, w329, w330, w321, w331, w332, w327, w326, w325) -> (w333:dbl[])
                    n183 = shared-variable "RT CompactRIO Target 2\\Library 1.lvlib\\Inject_Arrays"(w333) -> ()  [unwired: 1 in, 1 out]
                  }
                  frame #12 {
                    n184 = call-poly <vilib>:"Read From Spreadsheet File.vi"() -> ("all rows"=w336:dbl[][])  [unwired: 7 in, 4 out]
                    n185 = Reshape Array(w336, w335) -> (w334:dbl[])
                    "Lambda" <- w334
                    n186 = shared-variable "RT CompactRIO Target 2\\Library 1.lvlib\\Inject_Arrays_Lambda"(w334) -> ()  [unwired: 1 in, 1 out]
                  }
                }
              }
            }
            n187 = case shown="True" w252 {
              tunnel: w259 -> [_ w266]
              frame False {
              }
              frame True {
                n188 = flat-sequence {
                  tunnel: w266 -> [w269]
                  tunnel: [w269] -> w265
                  tunnel: w265 -> [w273]
                  frame #0 {
                    n189 = local write "Enum 1"(u16 1 ("Test number")) -> ()
                    "Test number" <- "Select Test Type"
                  }
                  frame #1 {
                    n190 = Enqueue Element(queue=w273, element=Control_3."main" ("Enum")) -> (queue out=w271:refnum<queue>)  [unwired: 2 in, 2 out]
                    n191 = property on="Stop Test" class="Bool (strict)"("DisabledEnum"=T11."Enabled" ("Disabled")) -> ()  [unwired: 2 in, 2 out]
                    n192 = Enqueue Element(queue=w271, element=Control_3."start test" ("Enum")) -> ()  [unwired: 2 in, 3 out]
                  }
                }
              }
            }
          }
        }
      }
      event "Log Test Data": Value Change {
        n193 = event-data() -> ()  [unwired: 1 in, 6 out]
        n194 = property on="File Name" class="Str (strict)"() -> ("Value"=w339:T5)  [unwired: 2 in, 2 out]
        n195 = String Length(string=w339) -> (length=w338:i32)
        n196 = Equal To 0?(x=w338) -> (x = 0?=w337:bool)
        n197 = case shown="True" w337 {
          frame False {
          }
          frame True {
            n198 = One Button Dialog(message="A filename has not been entered!") -> ()  [unwired: 1 in, 1 out]
          }
        }
      }
      event "Stop Test": Value Change {
        n199 = event-data() -> ()  [unwired: 1 in, 6 out]
        n200 = case shown="True" "Stop Test" {
          tunnel: w342 -> [_ w344]
          frame False {
          }
          frame True {
            n201 = flat-sequence {
              tunnel: w344 -> [w350]
              tunnel: [w350] -> w348
              tunnel: [w349] -> w347
              tunnel: w348 -> [w354]
              tunnel: [w353] -> w346
              tunnel: w347 -> [w353]
              tunnel: [w352] -> w345
              tunnel: w346 -> [w358]
              tunnel: w345 -> [w357]
              tunnel: [T11."Disabled and Grayed Out" ("Disabled")] -> _
              frame #0 {
                n202 = local read "Connected?"() -> (w349:bool)
                n203 = local write "Stop Cmd"(T1 1.0 ("Stop Cmd")) -> ()
              }
              frame #1 {
                n204 = Enqueue Element(queue=w354, element=Control_3."main" ("Enum")) -> (queue out=w352:refnum<queue>)  [unwired: 2 in, 2 out]
              }
              frame #2 {
                n205 = case shown="True" w358 {
                  tunnel: w357 -> [w359 w362]
                  tunnel: [w359 w361] -> _
                  frame False {
                  }
                  frame True {
                    n206 = local write "Connected?"(FALSE ("Connected?")) -> ()
                    n207 = Enqueue Element(queue=w362, element=Control_3."Multigas disconnect" ("Enum")) -> (queue out=w361:refnum<queue>)  [unwired: 2 in, 2 out]
                  }
                }
              }
            }
            n208 = local write "Start Test"(FALSE ("Start Test")) -> ()
          }
        }
      }
      event "Stopped?": Value Change {
        n209 = event-data() -> ()  [unwired: 1 in, 5 out]
        n210 = flat-sequence {
          tunnel: w366 -> [w370]
          tunnel: [w369] -> w365
          tunnel: [w368] -> w364
          tunnel: w365 -> [w372]
          tunnel: w364 -> [w371]
          frame #0 {
            n211 = local read "Connected?"() -> (w368:bool)
            n212 = Enqueue Element(queue=w370, element=Control_3."main" ("Enum")) -> (queue out=w369:refnum<queue>)  [unwired: 2 in, 2 out]
          }
          frame #1 {
            n213 = case shown="True" w371 {
              tunnel: w372 -> [_ w373]
              frame False {
              }
              frame True {
                n214 = local write "Connected?"(FALSE ("Connected?")) -> ()
                n215 = Enqueue Element(queue=w373, element=Control_3."Multigas disconnect" ("Enum")) -> ()  [unwired: 2 in, 3 out]
              }
            }
          }
        }
      }
      event "Alarm ack": Value Change {
        # "system alarm - set to off"
        n216 = event-data() -> ()  [unwired: 1 in, 5 out]
        n217 = local write "Acknowledge"(TRUE ("Acknowledge")) -> ()
        n218 = property on="Soft Alarm" class="Bool (strict)"("Value"=FALSE ("Acknowledge")) -> ()  [unwired: 2 in, 2 out]
        n219 = property on="Alarm ack" class="Bool"("DisabledEnum"=T11."Disabled and Grayed Out" ("Disabled")) -> ()  [unwired: 2 in, 2 out]
      }
      event "Purge System": Value Change {
        n220 = event-data() -> ()  [unwired: 1 in, 5 out]
        n221 = flat-sequence {
          tunnel: w380 -> [w382]
          tunnel: [w382] -> w379
          tunnel: w379 -> [w383]
          frame #0 {
            n222 = local write "Enum 1"(u16 4 ("Test number")) -> ()
          }
          frame #1 {
            n223 = Enqueue Element(queue=w383, element=Control_3."start test" ("Enum")) -> ()  [unwired: 2 in, 3 out]
          }
        }
      }
      event "Clear log": Value Change {
        n224 = event-data() -> ()  [unwired: 1 in, 5 out]
        n225 = local write "Table"(string[][] [] ("Table")) -> ()
      }
      event "Adv Settings": Value Change {
        # "To be updated"
        # "SO2 conc\nNOx conc\nCO conc\nHC conc\nBleed ratio N2\nBleed ratio CO2"
        n226 = event-data() -> ()  [unwired: 1 in, 6 out]
        n227 = call "Advanced settings MAX.vi"() -> ("output cluster"=→"output cluster":T2)  [unwired: 1 in]
      }
      event "Home": Value Change {
        w388 = FALSE
        n228 = event-data() -> ()  [unwired: 1 in, 6 out]
      }
      event "Performance": Value Change {
        w391 = FALSE
        n229 = event-data() -> ()  [unwired: 1 in, 6 out]
      }
      event "Ageing": Value Change {
        w395 = FALSE
        n230 = event-data() -> ()  [unwired: 1 in, 6 out]
      }
      event "System": Value Change {
        w399 = FALSE
        n231 = event-data() -> ()  [unwired: 1 in, 6 out]
      }
      event "MFC": Value Change {
        w403 = FALSE
        n232 = event-data() -> ()  [unwired: 1 in, 6 out]
      }
      event "Analyser": Value Change {
        w408 = FALSE
        n233 = event-data() -> ()  [unwired: 1 in, 6 out]
      }
      event "Alarm": Value Change {
        w411 = FALSE
        n234 = event-data() -> ()  [unwired: 1 in, 6 out]
      }
    }
    "stop 2" <- w69
    n235 = local write "Tab Control"(w67) -> ()
    n236 = case shown="False" w66 {
      tunnel: [w81 w89] -> w68
      tunnel: w67 -> [w81 _]
      tunnel: w65 -> [_ w89]
      tunnel: w64 -> [_ w88]
      tunnel: w63 -> [_ w87]
      tunnel: w62 -> [_ w86]
      tunnel: w61 -> [_ w85]
      tunnel: w60 -> [_ w84]
      tunnel: w59 -> [_ w83]
      tunnel: w58 -> [_ w82]
      tunnel: [w79 w88] -> w57
      tunnel: [w78 w87] -> w56
      tunnel: [w74 w86] -> w55
      tunnel: [w75 w85] -> w54
      tunnel: [w76 w84] -> w53
      tunnel: [w77 w83] -> w52
      tunnel: [w80 w82] -> w51
      tunnel: w50 -> [w79 _]
      tunnel: w49 -> [w78 _]
      tunnel: w48 -> [w80 _]
      tunnel: w47 -> [w77 _]
      tunnel: w46 -> [w76 _]
      tunnel: w45 -> [w75 _]
      tunnel: w44 -> [w74 _]
      frame False {
      }
      frame True {
      }
    }
    n237 = local write "MFC"(w53) -> ()
    n238 = local write "Home"(w57) -> ()
    n239 = local write "System"(w54) -> ()
    n240 = local write "Alarm"(w51) -> ()
    n241 = local write "Ageing"(w55) -> ()
    n242 = local write "Analyser"(w52) -> ()
    n243 = local write "Performance"(w56) -> ()
  }
  n244 = node-c288(nitl_modes."Discard missed periods, maintain original phase" ("Mode")) -> (w15:T12)  [unwired: 4 in]
  n245 = node-c288(i64 100 ("Period")) -> (w8:T12)  [unwired: 3 in]
  n246 = timed-loop {
    timing: w15 -> [_]
    timing-out: [_] -> w14
    shift-right: [w544] -> _
    shift-left: path "" -> [w512]
    shift-right: [w603] -> _
    shift-left: w9 -> [w637]
    shift-right: [w545] -> _
    shift-left: _ -> [w613]
    shift-right: [w593] -> _
    shift-left: w9 -> [w596]
    shift-right: [w594] -> _
    shift-left: w9 -> [w595]
    shift-right: [w536] -> _
    shift-left: 0 ("t") -> [w535]
    shift-right: [w526] -> _
    shift-left: _ -> [w515]
    shift-right: [w525] -> _
    shift-left: _ -> [w516]
    shift-right: [w524] -> _
    shift-left: _ -> [w517]
    shift-right: [w523] -> _
    shift-left: _ -> [w518]
    shift-right: [w522] -> _
    shift-left: _ -> [w519]
    shift-right: [w521] -> _
    shift-left: _ -> [w520]
    shift-right: [w502] -> _
    shift-left: _ -> [w503]
    stop <- w636 stop-if-true
    w552 = 54321.0 ("y")
    # "56 first gas"
    # "Flow Rate Guide"
    # "Temperature Guide"
    # "0   Flow Rate 1\n1   Flow Rate 2\n     ECM 1\n     ECM 2\n2   CO2 U\n3   CO U\n4   HC U\n5   O2 U\n7   CO2 D\n8   CO D\n9   HC D\n10 O2 D\n12 TC1X\n13 TC2A\n14 TC3Y\n15 TC4B\n16 TC5\n17 TC6\n32 Venturi 1\n33 Venturi 2\n34 Tank\n35 Bearing 1\n36 Bearing 2\n38 Ex A\n39 Ex B\n40 Ex C\n41 Ex D\n     MFC Box\n42 Furnace 1\n43 Furnace 2\n44 NO 1 ?? \n45 Lambda 1\n46 NO 2 ??\n47 Lambda 2\n56 CO (L)\n57 CO (H)\n58CO2\n59 O2\n60 THC\n61 NO\n62 NOx\n63 NO2"
    n247 = node-c288() -> (→"Finished Late? [i-1]":bool, →"Iteration Duration":i64)  [unwired: 1 in, 1 out]
    n248 = shared-variable "RT CompactRIO Target 2\\Library 1.lvlib\\DATA"() -> (w635:dbl[])  [unwired: 1 in, 1 out]
    n249 = local read "MKS"() -> (w433:bool)
    n250 = Type Cast(type=w635, x=w635) -> (*(type *) &x=w645:dbl[])
    n251 = local read "Advanced Logging"() -> (w549:bool)
    n252 = Delete From Array(array=w645, length=4, index=0) -> (deleted portion=w642:dbl[], array with subset deleted=w428:dbl[])
    n253 = call "MKS.vi"("IP Address"="192.168.254.1", "Connect"=w433) -> ("Emissions"=w513:dbl[])  [unwired: 9 in]
    n254 = call "MKS.vi"("IP Address"="192.168.254.2", "Connect"=FALSE) -> ("Emissions"=w514:dbl[])  [unwired: 9 in]
    n255 = local read "Full System"() -> (w543:bool)
    n256 = Index Array(array=w513, index=0) -> (element=w556:dbl)
    n257 = Index Array(array=w514, index=0) -> (element=w554:dbl)
    n258 = case shown="True" w549 {
      tunnel: [w741 w792] -> w550
      tunnel: w428 -> [w742 w792]
      tunnel: [w740 "Time\tFlow 1 g/s\tFlow 2 g/s\tECM 1\tECM 2\tTank Pressure\tTC1X\tTC2A\tTCY\tTC4B\tTC5\tTC6\tTC7\tTC8\tTC9\tTC10\tTC11\tTC12\tTC13\tTC14\tTC15\tTC16\tTC17\tTC18\tTC19\tTC20\tC Vent 1\tTC Vent 2\tTC Tank\tTC Fan B1\tTC Fan B2\tTC Cab\tTC Ex A\tTC Ex B\tTC Ex C\tTC Ex D\tSpare\tTC Furn 1\tTC Furn 2\tRapidox\tCO2 U %\tCO U %\tHC U ppm\tO2 U %\tNO U ppm\tCO2 D %\tCO D %\tHC D ppm\tO2 D %\tNO D ppm\tSwitch\tUEGO 1\tUEGO 2\tUEGO 3\tUEGO 4\tNOx Can 1\tNOx Can 2" ("Heading string 2")] -> w548
      tunnel: w543 -> [w739 _]
      frame False {
        n259 = case shown="True" w739 {
          tunnel: w742 -> [w757 w772]
          tunnel: [w748 w774] -> w741
          tunnel: ["Time\tFlow 1 g/s\tCO2 U %\tCO U %\tHC U ppm\tO2 U %\tNO U ppm\tCO2 D %\tCO D %\tHC D ppm\tO2 D %\tNO D ppm\tTC1X\tTC2A\tTCY\tTC4B\tTC5\tTC6\tTC7\tTC8\tRapidox\tLambda 1\tLambda 2\tNOX 1 ppm\tNOX 2 ppm\tUEGO 1\tUEGO 2" ("Heading string 2") "Time\tFlow 1 g/s\tFlow 2 g/s\tCO2 U %\tCO U %\tHC U ppm\tO2 U %\tNO U ppm\tCO2 D %\tCO D %\tHC D ppm\tO2 D %\tNO D ppm\tTC1X\tTC2A\tTCY\tTC4B\tTC5\tTC6\tTC7\tTC8\tRapidox\tLambda 1\tLambda 2\tNOX 1 ppm\tNOX 2 ppm\tUEGO 1\tUEGO 2" ("Heading string 2")] -> w740
          frame False {
            n260 = Delete From Array(array=w757, length=21, index=0) -> (deleted portion=w744:dbl[], array with subset deleted=w756:dbl[])
            n261 = Index Array(array=w756, index #1=47 ("index"), index #2=48 ("index"), index #3=49 ("index"), index #4=50 ("index"), index #5=51 ("index"), index #6=52 ("index"), index #7=53 ("index")) -> (element #1=w755:dbl, element #2=w754:dbl, element #3=w753:dbl, element #4=w752:dbl, element #5=w751:dbl, element #6=w750:dbl, element #7=w749:dbl)
            n262 = Delete From Array(array=w744, length=1, index=2) -> (array with subset deleted=w743:dbl[])  [unwired: 1 out]
            n263 = Build Array (concatenate)(w743, w755, w754, w753, w752, w751, w750, w749) -> (w748:dbl[])
          }
          frame True {
            n264 = Delete From Array(array=w772, length=21, index=0) -> (deleted portion=w769:dbl[], array with subset deleted=w773:dbl[])
            n265 = Index Array(array=w773, index #1=47 ("index"), index #2=48 ("index"), index #3=49 ("index"), index #4=50 ("index"), index #5=51 ("index"), index #6=52 ("index"), index #7=53 ("index")) -> (element #1=w781:dbl, element #2=w780:dbl, element #3=w779:dbl, element #4=w778:dbl, element #5=w777:dbl, element #6=w776:dbl, element #7=w775:dbl)
            n266 = Delete From Array(array=w769, length=2, index=1) -> (array with subset deleted=w767:dbl[])  [unwired: 1 out]
            n267 = Build Array (concatenate)(w767, w781, w780, w779, w778, w777, w776, w775) -> (w774:dbl[])
          }
        }
      }
      frame True {
        (unwired) "Time\tFlow 1 g/s\tFlow 2 g/s\tECM AFR\tCO2 U %\tCO U %\tHC U ppm\tO2 U %\tNO U ppm\tCO2 D %\tCO D %\tHC D ppm\tO2 D %\tNO D ppm\tTC1X\tTC2A\tTCY\tTC4B\tTC5\tTC6\tTC7\tTC8\tTC9\tTC10\tTC11\tTC12\tTC13\tTC14\tTC15\tTC16\tTC17\tTC18\tTC19\tTC20\tTC Vent 1\tTC Vent 2\tTC Fan B1\tTC Fan B2\tTC Cab\tTC Ex A\tTC Ex B\tTC Ex C\tTC Ex D\tTC Furn 1\tTC Furn 2\tNOX 1 ppm\tNLambda 1\tNOX 2 ppm\tNLambda 2\tEGO 1\tEGO 2\tEGO 3\tEGO 4\tCO2 U %\tCO U %\tHC U ppm\tO2 U %\tNO U ppm\tCO2 D %\tCO D %\tHC D ppm\tO2 D %\tNO D ppm\r\n" ("Heading string 2")
      }
    }
    n268 = Not Equal?(x=w556, y=w552) -> (x != y?=w555:bool)
    n269 = Not Equal?(x=w552, y=w554) -> (x != y?=w553:bool)
    n270 = Index Array(array=w642) -> (element #1=w545:dbl, element #2=w616:dbl, element #3=w431:dbl, element #4=w612:dbl)  [unwired: 4 in]
    "Error" <- w431
    "Test Loop" <- w545
    n271 = case shown="False" w555 {
      tunnel: [w798 w809] -> w416
      tunnel: w514 -> [w797 w808]
      tunnel: w513 -> [_ w807]
      tunnel: w553 -> [w796 w806]
      tunnel: [w795 w803] -> w551
      frame False {
        n272 = case shown="False" w796 {
          tunnel: [dbl[] [54321.0] w802] -> w798
          tunnel: w797 -> [_ w802]
          tunnel: ["\r\n" ("Heading string 2") "\tNO\tNO2 (150)\tNO2 (2000)\tN2O\tNH3 (300)\tNH3 (3000)\tHNCO (400)\tH2O\tCO2\tCO (500)\tCO (1)\tCH4 (250)\tCH4 (3000)\tNOxP\tPropane\r\n" ("Heading string 2")] -> w793
          frame False {
          }
          frame True {
          }
        }
        n273 = Build Array(" " ("Heading string 2"), w793) -> (w795:string[])
      }
      frame True {
        n274 = case shown="True" w806 {
          tunnel: [w811 w815] -> w809
          tunnel: w808 -> [_ w814]
          tunnel: w807 -> [w811 w813]
          tunnel: ["\rn" ("Heading string 2") "\tNO\tNO2 (150)\tNO2 (2000)\tN2O\tNH3 (300)\tNH3 (3000)\tHNCO (400)\tH2O\tCO2\tCO (500)\tCO (1)\tCH4 (250)\tCH4 (3000)\tNOxP\tPropane\r" ("Heading string 2")] -> w804
          frame False {
          }
          frame True {
            n275 = Build Array (concatenate)(w813, w814) -> (w815:dbl[])
          }
        }
        n276 = Build Array("\tNO\tNO2 (150)\tNO2 (2000)\tN2O\tNH3 (300)\tNH3 (3000)\tHNCO (400)\tH2O\tCO2\tCO (500)\tCO (1)\tCH4 (250)\tCH4 (3000)\tNOxP\tPropane" ("Heading string 2"), w804) -> (w803:string[])
      }
    }
    n277 = To Unsigned Long Integer(number=w612) -> (unsigned 32bit integer=w611:u32)
    n278 = Number To Boolean Array(number=w611) -> (Boolean array=w625:bool[])
    n279 = Index Array(array=w625) -> (element #2=w623:bool, element #3=w622:bool, element #4=w608:bool, element #5=→"ExtAnUp":bool, element #6=→"ExtAnDn":bool)  [unwired: 6 in, 1 out]
    "Extractor Fan On" <- w608
    n280 = case shown="0, Default" w616 {
      tunnel: [w835 TRUE FALSE] -> w615
      tunnel: [w836 FALSE TRUE] -> w614
      frame 0, Default {
        n281 = local read "Pass"() -> (w836:bool)
        n282 = local read "Fail"() -> (w835:bool)
      }
      frame 1 {
      }
      frame 2 {
      }
    }
    "Pass" <- w614
    "Fail" <- w615
    n283 = Or(x=w623, y=w622) -> (x .or. y?=→"Doors Open":bool)
    n284 = Not(x=w608) -> (.not. x?=→"Doors Unlocked":bool)
    n285 = Less?(x=w545, y=w613) -> (x < y?=w610:bool)
    n286 = Path To String(path="File Path") -> (string=w606:string)
    n287 = local read "Connected"() -> (w609:bool)
    n288 = Concatenate Strings(w606, "\\" ("string"), "File Name") -> (w559:string)
    n289 = call "Mexa_7170.vi"("String 1 In"=w519, "Connect"=FALSE, "connection ID 1 In"=w518, "error out 1 In"=w517, "connection ID 2 In"=w516, "error out 2 In"=w515, "Time In"=w520) -> ("Emissions"=→"Emissions":dbl[], "String 1 Out"=w522:string, "connection ID 1 Out"=w523:refnum<k5>, "error 1 out"=w524:errorcluster, "connection ID 2 Out"=w525:refnum<k16>, "Time Out"=w521:i16, "error 2 out"=w526:errorcluster)  [unwired: 2 in]
    n290 = And(x=w609, y=w610) -> (x .and. y?=w602:bool)
    n291 = local read "Mexa_One Emissions"() -> (w415:dbl[])
    n292 = call "Lambda Calc.vi"("Mexa In"=w415) -> ("Lambda Value"=w417:dbl)  [unwired: 10 in]
    n293 = Build Array (concatenate)(w415, w417, w416) -> (w418:dbl[])
    n294 = Insert Into Array(array=w428, index=53, new element=w418) -> (w427:dbl[])
    n295 = local write "Stopped?"(w602) -> ()
    n296 = Equal To 0?(x=w431) -> (x = 0?=w547:bool)
    n297 = Equal To 0?(x=w545) -> (x = 0?=w546:bool)
    n298 = Build Array (concatenate)(w550, w418) -> (w638:dbl[])
    n299 = Equal?(x=w545, y=2.0) -> (x = y?=w567:bool)
    n300 = String To Path(string=w559) -> (path=w604:path)
    n301 = Build Array(w547, w546) -> (w620:bool[])
    n302 = Equal?(x=w545, y=3.0) -> (x = y?=w564:bool)
    n303 = Equal?(x=w545, y=4.0) -> (x = y?=w562:bool)
    n304 = Boolean Array To Number(Boolean array=w620) -> (number=w619:u32)
    n305 = Index Array(array=w427, index=4) -> (element=→"Pressure":dbl)
    n306 = Not Equal?(x=w604, y=w512) -> (x != y?=w647:bool)
    n307 = Compound Arithmetic op=OR(w567, w564, w562) -> (w566:bool)
    n308 = case shown="1" w619 {
      tunnel: [w861 w862 w867 w869] -> _
      tunnel: [w861 w862 w867 w869] -> _
      tunnel: [w861 w862 w867 w869] -> w618
      tunnel: [w861 w862 w865 w869] -> w617
      tunnel: [T11."Enabled" ("Disabled") T11."Enabled" ("Disabled") w865 w869] -> _
      tunnel: [FALSE FALSE FALSE TRUE] -> w601
      frame 0, Default {
        w861 = T11."Disabled and Grayed Out" ("Disabled")
      }
      frame 1 {
        w862 = T11."Disabled and Grayed Out" ("Disabled")
      }
      frame 2 {
        w865 = T11."Enabled" ("Disabled")
        w867 = T11."Disabled and Grayed Out" ("Disabled")
      }
      frame 3 {
        w869 = T11."Enabled" ("Disabled")
        (unwired) T11."Disabled and Grayed Out" ("Disabled")
      }
    }
    n309 = local read "Log Test Data"() -> (w560:bool)
    n310 = for {
      tunnel: w638 -> [w877] mode=indexing
      tunnel: [w876] -> w649 mode=indexing
      n311 = Number To Fractional String(number=w877, precision (6)=i16 3) -> (F-format string=w876:string)  [unwired: 2 in]
    }
    n312 = Select(t=w604, s=w647, f=w512) -> (s? t:f=w648:path)
    n313 = And(x=w560, y=w566) -> (x .and. y?=w663:bool)
    "Log?" <- w663
    n314 = case shown="True" w647 {
      tunnel: w648 -> [w870 w875]
      tunnel: [w870 w874] -> w646
      tunnel: w551 -> [_ w872]
      tunnel: w548 -> [_ w871]
      frame False {
      }
      frame True {
        # "setting up the header"
        n315 = Build Array (concatenate)(w871, w872) -> (w873:string[])
        n316 = call-poly <vilib>:"Write To Spreadsheet File.vi"("1D data"=w873, "file path (dialog if empty)"=w875) -> ("new file path (Not A Path if cancelled)"=w874:path)  [unwired: 6 in]
      }
    }
    n317 = Equal?(x=w545, y=0.0) -> (x = y?=w590:bool)
    n318 = case shown="0, Default" w545 {
      tunnel: [w822 w824 w827 w828 TRUE FALSE] -> w442
      tunnel: [w822 w824 w827 TRUE w830 w833] -> w440
      tunnel: [TRUE w824 w827 w828 w830 w833] -> w439
      tunnel: [w822 TRUE TRUE w828 w830 w833] -> w424
      frame 0, Default {
        w822 = FALSE
      }
      frame 1 {
        w824 = FALSE
      }
      frame 2 {
        w827 = FALSE
      }
      frame 3 {
        w828 = FALSE
      }
      frame 4 {
        w830 = FALSE
        n319 = local write "Stop Cmd"(T1 0.0 ("Stop Cmd")) -> ()
      }
      frame 5 {
        w833 = FALSE
      }
    }
    n320 = property on="Compile Test Button" class="Bool"("DisabledEnum"=w618) -> ()  [unwired: 2 in, 2 out]
    n321 = property on="Purge System" class="Bool"("DisabledEnum"=w617) -> ()  [unwired: 2 in, 2 out]
    n322 = property class="VI"("Front Panel.Closeable"=w601) -> ()  [unwired: 2 in, 2 out]
    n323 = local read "Full System"() -> (w591:bool)
    n324 = Index Array(array=w418, index #1=0 ("index"), index #2=1 ("index"), index #3=2 ("index"), index #4=3 ("index")) -> ()  [unwired: 4 out]
    n325 = Equal?(x=w431, y=1024.0) -> (x = y?=w429:bool)
    n326 = case shown="True" "Demo On" {
      tunnel: w442 -> [w667 w671]
      tunnel: [w667 w670] -> w441
      tunnel: w440 -> [w669 _]
      tunnel: w439 -> [w668 _]
      tunnel: [w668 w670] -> w438
      tunnel: [w669 TRUE] -> w437
      tunnel: [w667 w671] -> w426
      tunnel: [w666 w670] -> w425
      tunnel: w424 -> [w666 _]
      frame False {
      }
      frame True {
        w670 = FALSE
      }
    }
    "Cool Down" <- w441
    "Test In Progress" <- w437
    "Standby" <- w438
    "Warm Up" <- w425
    n327 = case shown="False" w429 {
      tunnel: w431 -> [w664 _]
      tunnel: [w664 0.0 ("Numeric")] -> w432
      frame False {
      }
      frame True {
      }
    }
    n328 = Build Array(w591, w590) -> (w592:bool[])
    n329 = local write "Stop Test"(w426) -> ()
    n330 = Boolean Array To Number(Boolean array=w592) -> (number=w589:u32)
    n331 = call "Demo_Guide.vi"("Time In"=w503, "Temperature Sync"="Demo Sync", "Duration -1"="Duration -1", "TempGuide"="Demo On") -> ("Output array"=w478:dbl[], "Time out"=w502:i32)  [unwired: 6 in]
    n332 = Not Equal To 0?(x=w432) -> (x != 0?=w640:bool)
    n333 = Not Equal?(x=w432, y=w637) -> (x != y?=w639:bool)
    n334 = case shown="False" w663 {
      tunnel: w646 -> [w881 w889]
      tunnel: [w881 w901] -> w544
      tunnel: w649 -> [_ w897]
      tunnel: w596 -> [_ w890]
      tunnel: w595 -> [w880 w885]
      tunnel: [w880 w887] -> w594
      tunnel: [w879 w886] -> w593
      frame False {
        n335 = local read "Log interval (seconds)"() -> (w879:T1)
      }
      frame True {
        n336 = Get Date/Time In Seconds() -> (seconds since 1Jan1904=w898:timestamp)
        n337 = Decrement(x=w890) -> (x-1=w891:T1)
        n338 = Less Than 0?(x=w891) -> (x < 0?=w892:bool)
        n339 = Equal To 0?(x=w891) -> (x = 0?=w893:bool)
        n340 = Build Array(w892, w893) -> (w894:bool[])
        n341 = Path To String(path=w889) -> (string=w884:string)
        "File name" <- w884
        n342 = Format Date/Time String(time format string (%c)="%d/%m/%y %H:%M:%S", seconds (now)=w898) -> (date/time string=w899:string)  [unwired: 1 in]
        n343 = Boolean Array To Number(Boolean array=w894) -> (number=w895:u32)
        n344 = case shown="2" w895 {
          tunnel: w890 -> [w908 w909 _]
          tunnel: [w907 w909 w912] -> w886
          tunnel: w884 -> [w906 w911 w915]
          tunnel: [w903 w911 w913] -> w888
          tunnel: [w902 w910 w914] -> w887
          tunnel: w885 -> [w902 w910 w918]
          frame 0, Default {
            n345 = Number To Decimal String(number=w902) -> (decimal integer string=w904:string)  [unwired: 1 in]
            n346 = call <vilib>:"Space Constant.vi"() -> ("String"=w905:string)
            n347 = Decrement(x=w908) -> (x-1=w907:T1)
            n348 = Concatenate Strings(w906, w905, w904) -> (w903:string)
          }
          frame 1 {
          }
          frame 2 {
            n349 = Increment(x=w918) -> (x+1=w914:dbl)
            n350 = local read "Log interval (seconds)"() -> (w912:T1)
            n351 = Number To Decimal String(number=w914) -> (decimal integer string=w916:string)  [unwired: 1 in]
            n352 = call <vilib>:"Space Constant.vi"() -> ("String"=w917:string)
            n353 = Concatenate Strings(w915, w917, w916) -> (w913:string)
          }
        }
        n354 = Build Array (concatenate)(w899, w897) -> (w883:string[])
        n355 = String To Path(string=w888) -> (path=w882:path)
        n356 = call-poly <vilib>:"Write To Spreadsheet File.vi"("append to file? (new file:F)"=TRUE, "1D data"=w883, "file path (dialog if empty)"=w882) -> ("new file path (Not A Path if cancelled)"=w901:path)  [unwired: 5 in]
      }
    }
    n357 = And(x=w640, y=w639) -> (x .and. y?=w641:bool)
    n358 = Index Array(array=w427, index #1=0 ("index"), index #2=1 ("index"), index #3=56 ("index"), index #4=54 ("index"), index #5=42 ("index"), index #6=44 ("index"), index #7=45 ("index"), index #8=47 ("index"), index #9=57 ("index"), index #10=46 ("index"), index #11=5 ("index"), index #12=6 ("index"), index #13=7 ("index"), index #14=8 ("index"), index #15=9 ("index"), index #16=10 ("index"), index #17=25 ("index"), index #18=26 ("index"), index #19=27 ("index"), index #20=28 ("index"), index #21=29 ("index"), index #22=31 ("index"), index #23=32 ("index"), index #24=33 ("index"), index #25=34 ("index"), index #26=36 ("index"), index #27=37 ("index"), index #28=61 ("index"), index #29=62 ("index"), index #30=45 ("index"), index #31=46 ("index"), index #32=61 ("index"), index #33=3 ("index")) -> (element #1=w538:dbl, element #2=w537:dbl, element #3=w501:dbl, element #4=w499:dbl, element #5=w497:dbl, element #6=w496:dbl, element #7=w495:dbl, element #8=w494:dbl, element #9=w493:dbl, element #10=w491:dbl, element #11=w490:dbl, element #12=w488:dbl, element #13=w486:dbl, element #14=w484:dbl, element #15=w482:dbl, element #16=w480:dbl, element #17=w473:dbl, element #18=w471:dbl, element #19=w469:dbl, element #20=w467:dbl, element #21=w465:dbl, element #22=w463:dbl, element #23=w461:dbl, element #24=w459:dbl, element #25=w457:dbl, element #26=→"Furnace temp 1":dbl, element #27=→"Furnace temp 2":dbl, element #28=w455:dbl, element #29=w453:dbl, element #30=w451:dbl, element #31=w449:dbl, element #32=w447:dbl, element #33=w445:dbl)
    n359 = case shown="False" w641 {
      tunnel: w432 -> [w842 w854]
      tunnel: w639 -> [w845 _]
      tunnel: [w841 w854] -> w603
      frame False {
        n360 = Equal To 0?(x=w842) -> (x = 0?=w846:bool)
        n361 = And(x=w846, y=w845) -> (x .and. y?=w844:bool)
        n362 = case shown="True" w844 {
          frame False {
          }
          frame True {
            w849 = FALSE ("Ack hard alarm!")
            n363 = property on="Hard Alarm" class="Bool (strict)"("Value"=w849) -> ()  [unwired: 2 in, 2 out]
            n364 = property on="System Alarm" class="Bool (strict)"("Value"=w849) -> ()  [unwired: 2 in, 2 out]
            n365 = property on="System Alarm" class="Bool (strict)"("Value"=w849) -> ()  [unwired: 2 in, 2 out]
          }
        }
        n366 = case shown="True" "Acknowledge" {
          tunnel: [w847 0.0 ("Numeric")] -> w841
          tunnel: w842 -> [w847 _]
          frame False {
          }
          frame True {
          }
        }
      }
      frame True {
        n367 = local read "Table"() -> (w857:string[][])
        n368 = call "Error list.vi"("Error code"=w854, "Error array in"=w857) -> ("Hard alarm?"=w851:bool, "Error array out"=w856:string[][])  [unwired: 8 in]
        "Hard Alarm" <- w851
        n369 = Not(x=w851) -> (.not. x?=w852:bool)
        "Soft Alarm" <- w852
        n370 = Or(x=w852, y=w851) -> (x .or. y?=→"System Alarm":bool)
        n371 = case shown="True" w852 {
          frame False {
          }
          frame True {
            n372 = property on="Alarm ack" class="Bool"("DisabledEnum"=T11."Enabled" ("Disabled")) -> ()  [unwired: 2 in, 2 out]
          }
        }
        n373 = local write "Table"(w856) -> ()
        n374 = local write "Acknowledge"(FALSE ("Acknowledge")) -> ()
        n375 = property on="Tab Control" class="TabCtl (strict)"("Value"=6) -> ()  [unwired: 2 in, 2 out]
      }
    }
    n376 = case shown="1" w589 {
      tunnel: w538 -> [w817 w819 _ _]
      tunnel: w537 -> [_ w818 _ _]
      tunnel: [w817 w819 w820 w821] -> w477
      tunnel: [0.0 ("y") w818 w820 w821] -> w475
      frame 0, Default {
      }
      frame 1 {
      }
      frame 2 {
        w820 = 0.0 ("y")
      }
      frame 3 {
        w821 = 0.0 ("y")
      }
    }
    n377 = case shown="False" "Demo On" {
      tunnel: w501 -> [w703 _]
      tunnel: [w703 w735] -> w500
      tunnel: w499 -> [w702 _]
      tunnel: [w702 w705] -> w498
      tunnel: w497 -> [w701 _]
      tunnel: [w701 w712] -> _
      tunnel: w496 -> [w700 _]
      tunnel: [w700 w712] -> _
      tunnel: w495 -> [w699 _]
      tunnel: [w699 w712] -> _
      tunnel: w494 -> [w698 _]
      tunnel: [w698 w712] -> _
      tunnel: [w697 w733] -> w492
      tunnel: w493 -> [w697 _]
      tunnel: w491 -> [w696 _]
      tunnel: [w696 w712] -> _
      tunnel: w490 -> [w695 _]
      tunnel: [w695 w731] -> w489
      tunnel: w488 -> [w694 _]
      tunnel: [w694 w729] -> w487
      tunnel: w486 -> [w693 _]
      tunnel: [w693 w712] -> w485
      tunnel: w484 -> [w692 _]
      tunnel: [w692 w712] -> w483
      tunnel: w482 -> [w691 _]
      tunnel: [w691 w712] -> w481
      tunnel: w480 -> [w690 _]
      tunnel: [w690 w712] -> w479
      tunnel: w478 -> [_ w738]
      tunnel: w477 -> [w689 _]
      tunnel: [w689 w737] -> w476
      tunnel: w475 -> [w688 _]
      tunnel: [w688 w712] -> w474
      tunnel: w473 -> [w687 _]
      tunnel: [w687 w727] -> w472
      tunnel: w471 -> [w686 _]
      tunnel: [w686 w712] -> w470
      tunnel: w469 -> [w685 _]
      tunnel: [w685 w725] -> w468
      tunnel: w467 -> [w684 _]
      tunnel: [w684 w723] -> w466
      tunnel: w465 -> [w683 _]
      tunnel: [w683 w721] -> w464
      tunnel: w463 -> [w682 _]
      tunnel: [w682 w719] -> w462
      tunnel: w461 -> [w681 _]
      tunnel: [w681 w717] -> w460
      tunnel: w459 -> [w680 _]
      tunnel: [w680 w715] -> w458
      tunnel: w457 -> [w679 _]
      tunnel: [w679 w714] -> w456
      tunnel: w455 -> [w678 _]
      tunnel: [w678 w713] -> w454
      tunnel: w453 -> [w677 _]
      tunnel: [w677 w712] -> w452
      tunnel: w451 -> [w676 _]
      tunnel: [w676 w710] -> w450
      tunnel: w449 -> [w675 _]
      tunnel: [w675 w711] -> w448
      tunnel: w447 -> [w674 _]
      tunnel: [w674 w711] -> w446
      tunnel: w445 -> [w673 _]
      tunnel: [w673 w711] -> w444
      frame False {
      }
      frame True {
        w711 = 5.0 ("Numeric")
        w712 = 0.0 ("Numeric")
        n378 = Index Array(array=w738, index #1=2 ("index"), index #2=13 ("index"), index #3=14 ("index"), index #4=0 ("index"), index #5=1 ("index"), index #6=4 ("index"), index #7=5 ("index"), index #8=6 ("index"), index #9=7 ("index"), index #10=8 ("index"), index #11=9 ("index"), index #12=10 ("index"), index #13=11 ("index"), index #14=15 ("index"), index #15=3 ("index"), index #16=12 ("index")) -> (element #1=w737:dbl, element #2=w735:dbl, element #3=w733:dbl, element #4=w731:dbl, element #5=w729:dbl, element #6=w727:dbl, element #7=w725:dbl, element #8=w723:dbl, element #9=w721:dbl, element #10=w719:dbl, element #11=w717:dbl, element #12=w715:dbl, element #13=w714:dbl, element #14=w713:dbl, element #15=w710:dbl, element #16=w705:dbl)
      }
    }
    n379 = call "Flow_Guide-plot.vi"("Temperature Sync"="Flow Sync", "Temp Band % (e.g. 1%=1.01)"="Flow Band %", "Mean(Off)/Interval(On)"="Mean(Off)/Interval(On) 2", "Guide"="FlowGuide") -> ()  [unwired: 5 in, 3 out]
    n380 = Merge Signals(w492) -> (→"HC Concentration (ppm)":dynamicdata)
    n381 = Merge Signals(w472, w470, w468, w466, w464) -> (→"System Temperatures (°C)":dynamicdata)
    n382 = Merge Signals(w462, w460, w458, w456) -> (→"Heat Exchanger Temperatures (°C)":dynamicdata)
    n383 = Merge Signals(w454, w452) -> (→"NO Concentration (ppm)":dynamicdata)
    n384 = Merge Signals(w450, w448, w446, w444) -> (→"Lambda":dynamicdata)
    n385 = Merge Signals(w476, w474) -> (→"Flow Rate (g/s)":dynamicdata)
    n386 = Merge Signals(w500, w498) -> (→"O2/CO Concentration":dynamicdata)
    n387 = call "Temp_Guide-plot.vi"("Time In"=w535, "Temperature Sync"="Temperature Sync", "Temp Band % (e.g. 1%=1.01)"="Temp Band %", "Mean(Off)/Interval(On)"="Mean(Off)/Interval(On)", "TempGuide"="TempGuide") -> ("Graph 4"=w534:dbl, "Graph 3"=w533:dbl, "Graph 2"=w532:dbl, "Graph 1"=w531:dbl, "Time out"=w536:i32)  [unwired: 2 in]
    n388 = local read "stop 2"() -> (w636:bool)
    n389 = Merge Signals(w489, w487, w485, w483, w481, w479, w531, w532, w533, w534) -> (→"Sample Temperatures (°C)":dynamicdata)
    n390 = node-c288() -> ()  [unwired: 1 in, 1 out]
  }
  n391 = timed-loop {
    timing: w8 -> [_]
    timing-out: [_] -> w7
    shift-right: [w937] -> _
    shift-left: _ -> [w938]
    shift-right: [w936] -> _
    shift-left: _ -> [w928]
    shift-right: [w935] -> _
    shift-left: _ -> [w927]
    shift-right: [w934] -> _
    shift-left: _ -> [w929]
    shift-right: [w933] -> _
    shift-left: _ -> [w930]
    shift-right: [w932] -> _
    shift-left: _ -> [w931]
    stop <- _ stop-if-true
    n392 = node-c288() -> ()  [unwired: 1 in, 1 out]
    n393 = shared-variable "RT CompactRIO Target 2\\Library 1.lvlib\\DATA_2"() -> (w955:dbl[])  [unwired: 1 in, 1 out]
    n394 = local read "Test Loop"() -> (w923:dbl)
    n395 = local read "Mexa One"() -> (w926:bool)
    n396 = case shown="\"CO\", Default" "Graph 1 Box" {
      tunnel: [0 ("index") 1 ("index") 2 ("index") 3 ("index") 4 ("index") 5 ("index") 6 ("index") 7 ("index")] -> w956
      tunnel: [8 ("index") 9 ("index") 10 ("index") 11 ("index") 12 ("index") 13 ("index") 14 ("index") 15 ("index")] -> w963
      frame "CO", Default {
      }
      frame "HC Cycle 1" {
      }
      frame "Air Cycle 1" {
      }
      frame "NO" {
      }
      frame "Air Bal" {
      }
      frame "HC Bal" {
      }
      frame "Air Cycle 2" {
      }
      frame "HC Cycle 2" {
      }
    }
    n397 = case shown="\"Air Cycle 2\"" "Graph 2 Box" {
      tunnel: [0 ("index") 1 ("index") 2 ("index") 3 ("index") 4 ("index") 5 ("index") 6 ("index") 7 ("index")] -> w947
      tunnel: [8 ("index") 9 ("index") 10 ("index") 11 ("index") 12 ("index") 13 ("index") 14 ("index") 15 ("index")] -> w948
      frame "CO" {
      }
      frame "HC Cycle 1", Default {
      }
      frame "Air Cycle 1" {
      }
      frame "NO" {
      }
      frame "Air Bal" {
      }
      frame "HC Bal" {
      }
      frame "Air Cycle 2" {
      }
      frame "HC Cycle 2" {
      }
    }
    n398 = case shown="\"Air Cycle 1\", Default" "Graph 3 Box" {
      tunnel: [0 ("index") 1 ("index") 2 ("index") 3 ("index") 4 ("index") 5 ("index") 6 ("index") 7 ("index")] -> w945
      tunnel: [8 ("index") 9 ("index") 10 ("index") 11 ("index") 12 ("index") 13 ("index") 14 ("index") 15 ("index")] -> w946
      frame "CO" {
      }
      frame "HC Cycle 1" {
      }
      frame "Air Cycle 1", Default {
      }
      frame "NO" {
      }
      frame "Air Bal" {
      }
      frame "HC Bal" {
      }
      frame "Air Cycle 2" {
      }
      frame "HC Cycle 2" {
      }
    }
    n399 = case shown="\"NO\", Default" "Graph 4 Box" {
      tunnel: [0 ("index") 1 ("index") 2 ("index") 3 ("index") 4 ("index") 5 ("index") 6 ("index") 7 ("index")] -> w943
      tunnel: [8 ("index") 9 ("index") 10 ("index") 11 ("index") 12 ("index") 13 ("index") 14 ("index") 15 ("index")] -> w944
      frame "CO" {
      }
      frame "HC Cycle 1" {
      }
      frame "Air Cycle 1" {
      }
      frame "NO", Default {
      }
      frame "Air Bal" {
      }
      frame "HC Bal" {
      }
      frame "Air Cycle 2" {
      }
      frame "HC Cycle 2" {
      }
    }
    n400 = call "Mexa_One.vi"("String 1 In"=w931, "Connect"=w926, "connection ID 1 In"=w930, "error out 1 In"=w929, "connection ID 2 In"=w927, "error out 2 In"=w928, "Time In"=w938, "Test Loop"=w923) -> ("Emissions"=w925:dbl[], "String 1 Out"=w932:string, "connection ID 1 Out"=w933:refnum<k5>, "error 1 out"=w934:errorcluster, "connection ID 2 Out"=w935:refnum<k16>, "Time Out"=w937:i16, "error 2 out"=w936:errorcluster)  [unwired: 1 in]
    "Mexa_One Emissions" <- w925
    n401 = Index Array(array=w955, index #1=w956, index #2=w963) -> (element #1=w958:dbl, element #2=w957:dbl)
    n402 = Index Array(array=w955, index #1=w947, index #2=w948) -> (element #1=w954:dbl, element #2=w953:dbl)
    n403 = Index Array(array=w955, index #1=w945, index #2=w946) -> (element #1=w952:dbl, element #2=w951:dbl)
    n404 = Index Array(array=w955, index #1=w943, index #2=w944) -> (element #1=w950:dbl, element #2=w949:dbl)
    n405 = Merge Signals(w958, w957) -> (→"MFC Graph 1":dynamicdata)
    n406 = Merge Signals(w954, w953) -> (→"MFC Graph 2":dynamicdata)
    n407 = Merge Signals(w952, w951) -> (→"MFC Graph 3":dynamicdata)
    n408 = Merge Signals(w950, w949) -> (→"MFC Graph 4":dynamicdata)
    n409 = call "MKS.vi"("IP Address"="192.168.254.2" ("IP_ADD [127.0.0.1]"), "Connect"="MKS 5Hz") -> ("Emissions"=w924:dbl[])  [unwired: 9 in]
    n410 = Build Array (concatenate)(w955, w925, w924) -> (w968:dbl[])
    n411 = for {
      tunnel: w968 -> [w1049] mode=indexing
      tunnel: [w1048] -> w971 mode=indexing
      n412 = Number To Fractional String(number=w1049, precision (6)=i16 3) -> (F-format string=w1048:string)  [unwired: 2 in]
    }
    n413 = Get Date/Time In Seconds() -> (seconds since 1Jan1904=w974:timestamp)
    n414 = local read "File name"() -> (w978:string)
    n415 = Format Date/Time String(time format string (%c)="%d/%m/%y %H:%M:%S", seconds (now)=w974) -> (date/time string=w972:string)  [unwired: 1 in]
    n416 = Index Array(array=w924, index="HC Index") -> (element=→"MKS HC":dbl)
    n417 = Concatenate Strings(w978, "_MFC" ("string")) -> (w976:string)
    n418 = Build Array (concatenate)(w972, w971) -> (w970:string[])
    n419 = String To Path(string=w976) -> (path=w973:path)
    n420 = local read "Log?"() -> (w969:bool)
    n421 = case shown="True" w969 {
      tunnel: w973 -> [w1043 w1046]
      tunnel: [w1043 w1044] -> _
      tunnel: w970 -> [_ w1045]
      frame False {
      }
      frame True {
        n422 = call-poly <vilib>:"Write To Spreadsheet File.vi"("append to file? (new file:F)"=TRUE, "1D data"=w1045, "file path (dialog if empty)"=w1046) -> ("new file path (Not A Path if cancelled)"=w1044:path)  [unwired: 5 in]
      }
    }
    n423 = node-c288() -> ()  [unwired: 1 in, 1 out]
  }
  n424 = while {
    tunnel: w42 -> [w1057]
    tunnel: w26 -> [w1055]
    tunnel: w28 -> [w1054]
    tunnel: [FALSE ("stop 2")] -> w16
    stop <- w1058 stop-if-true
    n425 = Dequeue Element(queue=w1057) -> (element=w1056:T10)  [unwired: 2 in, 3 out]
    n426 = case shown="\"load cycle\"" w1056 {
      tunnel: w1055 -> [_ _ _ w1113 w1124 w1160 w1194 _ _ _ _ _ _ _ w1557 _ _ _ _ _ _ _ _]
      tunnel: w1054 -> [_ _ _ _ _ _ _ _ w1207 w1222 w1277 w1322 _ _ _ _ _ _ _ _ _ _ _]
      frame "main", Default {
        # "20"
        # "25"
        # "30"
        # "15"
        # "10"
        # "5"
        # "0"
        # "30"
        # "25"
        # "20"
        # "15"
        # "10"
        # "5"
        # "0"
        # "Output Cluster\n\n0 NOx Conc\n1 CO conc %\n2 HC conc %\n3 Bleed H2O \n4 Bleed CO2\n5 Bleed N2 \n6 lambda P\n7 lambda I\n8 lambda D\n9 purge duration\n10 Target furnace lambda\n11 HC reaction ct\n12 Full system\n13 Log interval\n14 MKS 1\n15 MKS 2"
        n427 = local read "output cluster"() -> (w1087:T2)
        n428 = Unbundle(w1087) -> ("NOx Concentration (ppm)"=w1074:T1, "CO concentration %"=w1073:T1, "HC concentration %"=w1072:T1, "Bleed H2O %"=w1071:T1, "Bleed CO2 %"=w1070:T1, "Bleed N2 %"=w1084:T1, "lambda P"=w1083:T1, "lambda I"=w1082:T1, "lambda D"=w1085:T1, "Purge duration (seconds)"=w1086:T1, "Target furnace lambda"=w1079:T1, "HC reaction constant"=w1078:T1, w1080:i16, "Log interval (HRS)"=→"Log interval (seconds)":T1, w1067:i16, w1066:i16, "Advanced Logging"=→"Advanced Logging":bool, "Cycle Length (Hours)"=w1065:T1, "Heat Load Control"=w1064:bool, w1062:T1[])
        n429 = local read "Test Flow Rate(g/s)"() -> (w1099:T1)
        n430 = local read "Test number"() -> (w1104:u16)
        n431 = local read "Inlet LAMBDA"() -> (w1091:T1)
        n432 = local read "NO ppm Loff"() -> (w1089:T1)
        n433 = local read "NO:CO Ratio"() -> (w1088:T1)
        n434 = local read "Inlet O2 (%)"() -> (w1090:T1)
        n435 = local read "Connected"() -> (w1093:bool)
        n436 = Boolean To (0,1)(Boolean=w1064) -> (0, 1=w1063:i16)
        n437 = Boolean To (0,1)(Boolean=w1093) -> (0, 1=w1077:i16)
        n438 = Build Array (concatenate)("Stop Cmd", w1104, w1099, "Test Start Temperature (°C)", "Test Stop temperature (°C)", "Furnace Ramp Rate (°C/min)", w1091, w1090, "Inlet LAMBDA Rich", "Inlet LAMBDA Lean", "Inlet Temperature (°C)", "NO ppm SW", w1089, w1088, "Temperature Limit (°C)", w1077, "Inlet temp Age", "Flow rate Age", w1074, w1073, w1072, w1071, w1070, w1084, w1083, w1082, w1085, w1086, w1079, w1078, w1080, w1065, w1063, w1062) -> (w1095:T1[])
        n439 = Not Equal To 0?(x=w1080) -> (x != 0?=→"Full System":bool)
        n440 = shared-variable "RT CompactRIO Target 2\\Library 1.lvlib\\Control Variables"(w1095) -> ()  [unwired: 1 in, 1 out]
        n441 = Not Equal To 0?(x=w1067) -> (x != 0?=w1068:bool)
        "Mexa One" <- w1068
        n442 = Not Equal To 0?(x=w1066) -> (x != 0?=w1061:bool)
        "MKS" <- w1061
        n443 = Or(x=w1068, y=w1061) -> (x .or. y?=→"Connected":bool)
      }
      frame "start test" {
        w1105 = FALSE
        n444 = property on="Pass" class="Bool (strict)"("Value"=w1105) -> ()  [unwired: 2 in, 2 out]
        n445 = property on="Fail" class="Bool (strict)"("Value"=w1105) -> ()  [unwired: 2 in, 2 out]
        n446 = local write "Pass"(w1105) -> ()
        n447 = local write "Fail"(w1105) -> ()
        n448 = shared-variable "RT CompactRIO Target 2\\Library 1.lvlib\\Enum 1"("Enum 1") -> ()  [unwired: 1 in, 1 out]
      }
      frame "clear table 1" {
        n449 = property on="Sub-Cycle Name" class="Str (strict)"("Value"="" ("Subcycle name")) -> ()  [unwired: 2 in, 2 out]
        n450 = local write "Flag1"(FALSE) -> ()
        n451 = local write "Sub-Cycle Pattern"(string[][] [["", "0", "", "", "", "", "", "", "", "", "", "", ""], ["", "", "", "", "", "", "", "", "", "", "", "", ""], ["", "", "", "", "", "", "", "", "", "", "", "", ""], ["", "", "", "", "", "", "", "", "", "", "", "", ""], ["", "", "", "", "", "", "", "", "", "", "", "", ""], ["", "", "", "", "", "", "", "", "", "", "", "", ""], ["", "", "", "", "", "", "", "", "", "", "", "", ""], ["", "", "", "", "", "", "", "", "", "", "", "", ""], ["", "", "", "", "", "", "", "", "", "", "", "", ""], ["", "", "", "", "", "", "", "", "", "", "", "", ""], ["", "", "", "", "", "", "", "", "", "", "", "", ""], ["", "", "", "", "", "", "", "", "", "", "", "", ""], ["", "", "", "", "", "", "", "", "", "", "", "", ""], ["", "", "", "", "", "", "", "", "", "", "", "", ""], ["", "", "", "", "", "", "", "", "", "", "", "", ""], ["", "", "", "", "", "", "", "", "", "", "", "", ""], ["", "", "", "", "", "", "", "", "", "", "", "", ""], ["", "", "", "", "", "", "", "", "", "", "", "", ""], ["", "", "", "", "", "", "", "", "", "", "", "", ""], ["", "", "", "", "", "", "", "", "", "", "", "", ""], ["", "", "", "", "", "", "", "", "", "", "", "", ""], ["", "", "", "", "", "", "", "", "", "", "", "", ""], ["", "", "", "", "", "", "", "", "", "", "", "", ""], ["", "", "", "", "", "", "", "", "", "", "", "", ""], ["", "", "", "", "", "", "", "", "", "", "", "", ""], ["", "", "", "", "", "", "", "", "", "", "", "", ""], ["", "", "", "", "", "", "", "", "", "", "", "", ""], ["", "", "", "", "", "", "", "", "", "", "", "", ""], ["", "", "", "", "", "", "", "", "", "", "", "", ""], ["", "", "", "", "", "", "", "", "", "", "", "", ""], ["", "", "", "", "", "", "", "", "", "", "", "", ""]]) -> ()
      }
      frame "update list 1" {
        n452 = String To Path(string=w1113) -> (path=w1112:path)
        n453 = List Folder(path=w1112, pattern="*.eyes") -> (filenames=w1111:string[])  [unwired: 2 in, 3 out]
        n454 = property on="Sub-Cycle List" class="LstBox (strict)"("Item Names"=w1111) -> ()  [unwired: 2 in, 2 out]
      }
      frame "save subc" {
        w1117 = ".eyes" ("string")
        n455 = local read "Sub-Cycle Name"() -> (w1116:T5)
        n456 = String To Path(string=w1124) -> (path=w1129:path)
        n457 = Equal?(x=w1116, y="") -> (x = y?=w1121:bool)
        n458 = List Folder(path=w1129, pattern="*.eyes" ("string")) -> (filenames=w1128:string[])  [unwired: 2 in, 3 out]
        n459 = Concatenate Strings(w1116, w1117) -> (w1115:string)
        n460 = Concatenate Strings(w1124, w1116, w1117) -> (w1130:string)
        n461 = Search 1D Array(1D array=w1128, element=w1115) -> (index of element=w1127:i32)  [unwired: 1 in]
        n462 = case shown="True" w1121 {
          tunnel: [TRUE FALSE] -> w1120
          frame False {
          }
          frame True {
            n463 = One Button Dialog(message="Insert file name!") -> ()  [unwired: 1 in, 1 out]
          }
        }
        n464 = String To Path(string=w1130) -> (path=w1123:path)
        n465 = Equal?(x=w1127, y=-1) -> (x = y?=w1125:bool)
        n466 = case shown="False" w1125 {
          selector: w1125 -> [_ w1136]
          tunnel: [w1134 w1136] -> w1119
          frame False {
            n467 = Two Button Dialog(message="A file with this name already exists!\nDo you want to overwrite?") -> (T button?=w1134:bool)  [unwired: 2 in]
          }
          frame True {
          }
        }
        n468 = And(x=w1119, y=w1120) -> (x .and. y?=w1118:bool)
        n469 = case shown="True" w1118 {
          tunnel: w1123 -> [_ w1141]
          frame False {
          }
          frame True {
            n470 = local read "Sub-Cycle Pattern"() -> (w1140:string[][])
            n471 = call "Table check.vi"("Input table"=w1140) -> ("Incomplete?"=w1138:bool, "Length"=w1139:i32)  [unwired: 9 in]
            n472 = case shown="False" w1138 {
              tunnel: w1140 -> [w1149 _]
              tunnel: w1141 -> [w1148 _]
              tunnel: w1139 -> [w1147 _]
              tunnel: string[] [] -> [w1146 _]
              frame False {
                n473 = for {
                  N: w1147 -> [_]
                  tunnel: w1149 -> [w1156]
                  shift-right: [w1153] -> w1145
                  shift-left: w1146 -> [w1154]
                  i -> [w1155]
                  n474 = Index Array(array=w1156, index (row)=w1155) -> (element=w1152:string[])  [unwired: 1 in]
                  n475 = Delete From Array(array=w1152, index=0) -> (array with subset deleted=w1151:string[])  [unwired: 1 in, 1 out]
                  n476 = Build Array (concatenate)(w1154, w1151) -> (w1153:string[])
                }
                n477 = Build Array (concatenate)("SubCycle Data File for EYECAT - do not modify", w1145) -> (w1143:string[])
                n478 = call-poly <vilib>:"Write To Spreadsheet File.vi"("1D data"=w1143, "file path (dialog if empty)"=w1148) -> ()  [unwired: 6 in, 1 out]
              }
              frame True {
                n479 = One Button Dialog(message="The table is incomplete!\nplease review and save again!") -> ()  [unwired: 1 in, 1 out]
              }
            }
            n480 = local write "Flag1"(FALSE) -> ()
          }
        }
      }
      frame "load subc" {
        n481 = local read "Flag1"() -> (w1161:bool)
        n482 = case shown="True" w1161 {
          tunnel: [w1188 w1190] -> w1159
          tunnel: w1160 -> [w1188 w1190]
          tunnel: [TRUE w1189] -> w1158
          frame False {
          }
          frame True {
            n483 = Two Button Dialog(message="The table has been modified.\nDo you want to continue?") -> (T button?=w1189:bool)  [unwired: 2 in]
          }
        }
        n484 = case shown="True" w1158 {
          tunnel: w1159 -> [_ w1165]
          frame False {
          }
          frame True {
            n485 = property on="Sub-Cycle List" class="LstBox (strict)"() -> ("Item Names"=w1177:string[])  [unwired: 2 in, 2 out]
            n486 = Index Array(array=w1177, index="Sub-Cycle List") -> (element=w1164:string)
            n487 = Concatenate Strings(w1165, w1164) -> (w1175:string)
            n488 = Search/Split String(string=w1164, search string/char (-)=".") -> (substring before match=w1162:string)  [unwired: 1 in, 2 out]
            n489 = local write "Sub-Cycle Name"(w1162) -> ()
            n490 = String To Path(string=w1175) -> (path=w1174:path)
            n491 = call-poly <vilib>:"Read From Spreadsheet File.vi"("file path (dialog if empty)"=w1174) -> ("first row"=w1170:string[])  [unwired: 6 in, 4 out]
            n492 = Delete From Array(array=w1170, length=1, index=0) -> (array with subset deleted=w1167:string[])  [unwired: 1 out]
            n493 = Array Size(array=w1167) -> (size(s)=w1173:i32)
            n494 = Divide(x=w1173, y=12) -> (x/y=w1166:dbl)
            n495 = for {
              N: w1166 -> [_]
              shift-right: [w1183] -> _
              shift-left: w1167 -> [w1186]
              tunnel: [w1182] -> w1171 mode=indexing
              i -> [w1181]
              n496 = Increment(x=w1181) -> (x+1=w1180:i32)
              n497 = Delete From Array(array=w1186, length=12, index=0) -> (deleted portion=w1178:string[], array with subset deleted=w1183:string[])
              n498 = Number To Decimal String(number=w1180) -> (decimal integer string=w1179:string)  [unwired: 1 in]
              n499 = Build Array (concatenate)(w1179, w1178) -> (w1182:string[])
            }
            n500 = local write "Sub-Cycle Pattern"(w1171) -> ()
          }
        }
      }
      frame "delete subc" {
        n501 = Two Button Dialog(message="This operation will permanently delete this file!\nDo you want to continue?") -> (T button?=w1193:bool)  [unwired: 2 in]
        n502 = case shown="True" w1193 {
          tunnel: w1194 -> [_ w1199]
          frame False {
          }
          frame True {
            n503 = local read "Sub-Cycle List"() -> (w1196:i32)
            n504 = property on="Sub-Cycle List" class="LstBox (strict)"() -> ("Item Names"=w1197:string[])  [unwired: 2 in, 2 out]
            n505 = Index Array(array=w1197, index=w1196) -> (element=w1201:string)
            n506 = Concatenate Strings(w1199, w1201) -> (w1200:string)
            n507 = local write "Flag1"(FALSE) -> ()
            n508 = String To Path(string=w1200) -> (path=w1198:path)
            n509 = Delete(path (use dialog)=w1198) -> ()  [unwired: 4 in, 3 out]
          }
        }
      }
      frame "clear table 2" {
        n510 = property on="Cycle Name" class="Str (strict)"("Value"="" ("Subcycle name")) -> ()  [unwired: 2 in, 2 out]
        n511 = local write "Flag 2"(FALSE) -> ()
        n512 = local write "Cycle Pattern"(string[][] [["", "", "", "", ""], ["", "", "", "", ""], ["", "", "", "", ""], ["", "", "", "", ""], ["", "", "", "", ""], ["", "", "", "", ""], ["", "", "", "", ""], ["", "", "", "", ""], ["", "", "", "", ""], ["", "", "", "", ""], ["", "", "", "", ""], ["", "", "", "", ""], ["", "", "", "", ""], ["", "", "", "", ""], ["", "", "", "", ""], ["", "", "", "", ""], ["", "", "", "", ""], ["", "", "", "", ""], ["", "", "", "", ""], ["", "", "", "", ""], ["", "", "", "", ""], ["", "", "", "", ""], ["", "", "", "", ""], ["", "", "", "", ""], ["", "", "", "", ""], ["", "", "", "", ""], ["", "", "", "", ""], ["", "", "", "", ""], ["", "", "", "", ""], ["", "", "", "", ""], ["", "", "", "", ""]]) -> ()
      }
      frame "update list 2" {
        n513 = String To Path(string=w1207) -> (path=w1208:path)
        n514 = List Folder(path=w1208, pattern="*.eyec") -> (filenames=w1206:string[])  [unwired: 2 in, 3 out]
        n515 = property on="Cycle List" class="LstBox (strict)"("Item Names"=w1206) -> ()  [unwired: 2 in, 2 out]
      }
      frame "save cycle" {
        w1209 = ".eyec" ("string")
        n516 = local read "Cycle Name"() -> (w1210:T5)
        n517 = String To Path(string=w1222) -> (path=w1223:path)
        n518 = List Folder(path=w1223, pattern="*.eyec" ("string")) -> (filenames=w1221:string[])  [unwired: 2 in, 3 out]
        n519 = Equal?(x=w1210, y="") -> (x = y?=w1216:bool)
        n520 = Concatenate Strings(w1210, w1209) -> (w1212:string)
        n521 = Search 1D Array(1D array=w1221, element=w1212) -> (index of element=w1220:i32)  [unwired: 1 in]
        n522 = Concatenate Strings(w1222, w1210, w1209) -> (w1225:string)
        n523 = case shown="True" w1216 {
          tunnel: [TRUE FALSE] -> w1214
          frame False {
          }
          frame True {
            n524 = One Button Dialog(message="Insert file name!") -> ()  [unwired: 1 in, 1 out]
          }
        }
        n525 = String To Path(string=w1225) -> (path=w1224:path)
        n526 = Equal?(x=w1220, y=-1) -> (x = y?=w1218:bool)
        n527 = case shown="False" w1218 {
          selector: w1218 -> [_ w1274]
          tunnel: [w1272 w1274] -> w1215
          frame False {
            n528 = Two Button Dialog(message="A file with this name already exists!\nDo you want to overwrite?") -> (T button?=w1272:bool)  [unwired: 2 in]
          }
          frame True {
          }
        }
        n529 = And(x=w1215, y=w1214) -> (x .and. y?=w1213:bool)
        n530 = case shown="True" w1213 {
          tunnel: w1224 -> [_ w1232]
          frame False {
          }
          frame True {
            n531 = local read "Cycle Pattern"() -> (w1231:string[][])
            n532 = call "Table check.vi"("Input table"=w1231) -> ("Incomplete?"=w1229:bool, "Length"=w1230:i32)  [unwired: 9 in]
            n533 = case shown="False" w1229 {
              tunnel: w1232 -> [w1241 _]
              tunnel: w1231 -> [w1240 _]
              tunnel: w1230 -> [w1233 _]
              frame False {
                n534 = Number To Decimal String(number=w1233) -> (decimal integer string=w1236:string)  [unwired: 1 in]
                n535 = for {
                  N: w1233 -> [_]
                  tunnel: w1240 -> [w1270]
                  shift-right: [w1258] -> w1237
                  shift-left: string[] [] -> [w1268]
                  i -> [w1269]
                  w1249 = 12 ("length")
                  n536 = Index Array(array=w1270, index (row)=w1269) -> (element=w1264:string[])  [unwired: 1 in]
                  n537 = Index Array(array=w1264, index=3) -> (element=w1254:string)
                  n538 = Index Array(array=w1264, index=1) -> (element=w1253:string)
                  n539 = Concatenate Strings("C:\\Setup Files\\Subcycles Folder\\", w1253) -> (w1265:string)
                  n540 = String To Path(string=w1265) -> (path=w1266:path)
                  n541 = call-poly <vilib>:"Read From Spreadsheet File.vi"("file path (dialog if empty)"=w1266) -> ("first row"=w1257:string[])  [unwired: 6 in, 4 out]
                  n542 = Delete From Array(array=w1257, length=1, index=0) -> (array with subset deleted=w1251:string[])  [unwired: 1 out]
                  n543 = String Length(string=w1251) -> (length=w1260:i32[])
                  n544 = Array Size(array=w1260) -> (size(s)=w1252:i32)
                  n545 = Divide(x=w1252, y=w1249) -> (x/y=w1250:dbl)
                  n546 = Decrement(x=w1250) -> (x-1=w1242:dbl)
                  n547 = Multiply(x=w1249, y=w1242) -> (x*y=w1248:dbl)
                  n548 = Number To Decimal String(number=w1242) -> (decimal integer string=w1259:string)  [unwired: 1 in]
                  n549 = Delete From Array(array=w1251, length=12, index=w1248) -> (deleted portion=w1245:string[], array with subset deleted=w1246:string[])
                  n550 = Index Array(array=w1245, index=0) -> (element=w1243:string)
                  n551 = Build Array (concatenate)(w1253, w1254, w1259, w1243, w1246) -> (w1263:string[])
                  n552 = Build Array (concatenate)(w1268, w1263) -> (w1258:string[])
                }
                n553 = local write "Flag 2"(FALSE) -> ()
                n554 = Build Array (concatenate)("Cycle Data File for EYECAT - do not modify", w1236, w1237) -> (w1238:string[])
                n555 = call-poly <vilib>:"Write To Spreadsheet File.vi"("1D data"=w1238, "file path (dialog if empty)"=w1241) -> ()  [unwired: 6 in, 1 out]
              }
              frame True {
                n556 = One Button Dialog(message="The table is incomplete!\nplease review and save again!") -> ()  [unwired: 1 in, 1 out]
              }
            }
          }
        }
      }
      frame "load cycle" {
        n557 = local read "Flag 2"() -> (w1278:bool)
        n558 = case shown="True" w1278 {
          tunnel: [w1317 w1319] -> w1275
          tunnel: w1277 -> [w1317 w1319]
          tunnel: [TRUE ("T button?") w1318] -> w1276
          frame False {
          }
          frame True {
            n559 = Two Button Dialog(message="The table has been modified.\nDo you want to continue?") -> (T button?=w1318:bool)  [unwired: 2 in]
          }
        }
        n560 = case shown="True" w1276 {
          tunnel: w1275 -> [_ w1281]
          frame False {
          }
          frame True {
            n561 = property on="Cycle List" class="LstBox (strict)"() -> ("Item Names"=w1297:string[])  [unwired: 2 in, 2 out]
            n562 = Index Array(array=w1297, index="Cycle List") -> (element=w1283:string)
            n563 = Concatenate Strings(w1281, w1283) -> (w1296:string)
            n564 = Search/Split String(string=w1283, search string/char (-)=".") -> (substring before match=w1282:string)  [unwired: 1 in, 2 out]
            n565 = String To Path(string=w1296) -> (path=w1295:path)
            n566 = local write "Cycle Name"(w1282) -> ()
            n567 = call-poly <vilib>:"Read From Spreadsheet File.vi"("file path (dialog if empty)"=w1295) -> ("first row"=w1279:string[])  [unwired: 6 in, 4 out]
            n568 = Delete From Array(array=w1279, length=2, index=0) -> (array with subset deleted=w1280:string[])  [unwired: 1 out]
            n569 = Index Array(array=w1279, index=1) -> (element=w1294:string)
            n570 = Decimal String To Number(string=w1294) -> (number=w1293:i32)  [unwired: 2 in, 1 out]
            n571 = for {
              N: w1293 -> [_]
              tunnel: w1280 -> [w1315]
              tunnel: [w1310] -> w1288 mode=indexing
              shift-right: [w1300] -> _
              shift-left: 0 ("x") -> [w1301]
              i -> [w1314]
              w1311 = ""
              n572 = Increment(x=w1301) -> (x+1=w1299:i32)
              n573 = Increment(x=w1299) -> (x+1=w1307:i32)
              n574 = Increment(x=w1314) -> (x+1=w1309:i32)
              n575 = Number To Decimal String(number=w1309) -> (decimal integer string=w1308:string)  [unwired: 1 in]
              n576 = Index Array(array=w1315, index #1=w1301, index #2=w1299, index #3=w1307) -> (element #1=w1313:string, element #2=w1312:string, element #3=w1306:string)
              n577 = Build Array(w1308, w1313, w1311, w1312, w1311) -> (w1310:string[])
              n578 = Decimal String To Number(string=w1306) -> (number=w1305:i32)  [unwired: 2 in, 1 out]
              n579 = Multiply(x=w1305, y=12 ("x")) -> (x*y=w1303:i32)
              n580 = Compound Arithmetic op=ADD(w1303, 4, w1301) -> (w1300:i32)
            }
            n581 = Insert Into Array(array=string[][] [["", "", "", "", ""], ["", "", "", "", ""], ["", "", "", "", ""], ["", "", "", "", ""], ["", "", "", "", ""], ["", "", "", "", ""], ["", "", "", "", ""], ["", "", "", "", ""], ["", "", "", "", ""], ["", "", "", "", ""], ["", "", "", "", ""], ["", "", "", "", ""], ["", "", "", "", ""], ["", "", "", "", ""], ["", "", "", "", ""], ["", "", "", "", ""], ["", "", "", "", ""], ["", "", "", "", ""], ["", "", "", "", ""], ["", "", "", "", ""], ["", "", "", "", ""], ["", "", "", "", ""], ["", "", "", "", ""], ["", "", "", "", ""], ["", "", "", "", ""], ["", "", "", "", ""], ["", "", "", "", ""], ["", "", "", "", ""], ["", "", "", "", ""], ["", "", "", "", ""], ["", "", "", "", ""]], index (row)=0, new element=w1288) -> (w1287:string[][])  [unwired: 1 in]
            n582 = local write "Cycle Pattern"(w1287) -> ()
          }
        }
      }
      frame "delete cycle" {
        n583 = Two Button Dialog(message="This operation will permanently delete this file!\nDo you want to continue?") -> (T button?=w1323:bool)  [unwired: 2 in]
        n584 = case shown="True" w1323 {
          tunnel: w1322 -> [_ w1328]
          frame False {
          }
          frame True {
            n585 = local read "Cycle List"() -> (w1329:i32)
            n586 = property on="Cycle List" class="LstBox (strict)"() -> ("Item Names"=w1330:string[])  [unwired: 2 in, 2 out]
            n587 = Index Array(array=w1330, index=w1329) -> (element=w1327:string)
            n588 = Concatenate Strings(w1328, w1327) -> (w1326:string)
            n589 = String To Path(string=w1326) -> (path=w1325:path)
            n590 = Delete(path (use dialog)=w1325) -> ()  [unwired: 4 in, 3 out]
            n591 = local write "Flag 2"(FALSE) -> ()
          }
        }
      }
      frame "calc HC CO" {
        n592 = local read "Sub-Cycle Pattern"() -> (w1347:string[][])
        n593 = Index Array(array=w1347, index (col) #1=3 ("disabled index (col)"), index (col) #2=4 ("index (col)"), index (col) #3=11 ("index (col)")) -> (element #1=w1337:string[], element #2=w1344:string[], element #3=w1331:string[])  [unwired: 3 in]
        n594 = Array Size(array=w1337) -> (size(s)=w1335:i32)
        n595 = Search 1D Array(1D array=w1337, element="") -> (index of element=w1334:i32)  [unwired: 1 in]
        n596 = Equal?(x=w1334, y=-1) -> (x = y?=w1336:bool)
        n597 = Select(t=w1335, s=w1336, f=w1334) -> (s? t:f=w1333:i32)
        n598 = for {
          N: w1333 -> [_]
          tunnel: [w1358] -> w1341 mode=indexing
          tunnel: [w1357] -> w1340 mode=indexing
          tunnel: w1337 -> [w1356] mode=indexing
          tunnel: w1344 -> [w1355] mode=indexing
          tunnel: w1331 -> [w1354] mode=indexing
          w1353 = ""
          n599 = Not Equal?(x=w1356, y=w1353) -> (x != y?=w1352:bool)
          n600 = Not Equal?(x=w1355, y=w1353) -> (x != y?=w1351:bool)
          n601 = Not Equal?(x=w1354, y=w1353) -> (x != y?=w1350:bool)
          n602 = Compound Arithmetic op=AND(w1352, w1351, w1350) -> (w1349:bool)
          n603 = case shown="True" w1349 {
            tunnel: w1356 -> [_ w1387]
            tunnel: w1355 -> [_ w1386]
            tunnel: [w1359 w1383] -> w1357
            tunnel: [w1359 w1382] -> w1358
            tunnel: w1354 -> [_ w1360]
            frame False {
              w1359 = ""
            }
            frame True {
              # "O2Eq"
              n604 = Fract/Exp String To Number(string=w1360) -> (number=w1361:dbl)  [unwired: 3 in, 1 out]
              n605 = Fract/Exp String To Number(string=w1387) -> (number=w1368:dbl)  [unwired: 3 in, 1 out]
              n606 = Fract/Exp String To Number(string=w1386) -> (number=w1364:dbl)  [unwired: 3 in, 1 out]
              n607 = Decrement(x=w1368) -> (x-1=w1369:dbl)
              n608 = Divide(x=w1361, y=20000.0) -> (x/y=w1362:dbl)
              n609 = Multiply(x=4.76, y=w1368) -> (x*y=w1373:dbl)
              n610 = Multiply(x=w1369, y=100.0) -> (x*y=w1371:dbl)
              n611 = Add(x=w1364, y=w1362) -> (x+y=w1365:dbl)
              n612 = Add(x=0.33, y=w1373) -> (x+y=w1375:dbl)
              n613 = Divide(x=w1371, y=w1375) -> (x/y=w1376:dbl)
              n614 = Subtract(x=w1365, y=w1376) -> (x-y=w1378:dbl)
              n615 = Multiply(x=w1378, y=2.0) -> (x*y=w1366:dbl)
              n616 = Divide(x=w1378, y=5.0) -> (x/y=w1367:dbl)
              n617 = Number To Fractional String(number=w1367, width (-)=i16 6, precision (6)=i16 3) -> (F-format string=w1382:string)  [unwired: 1 in]
              n618 = Number To Fractional String(number=w1366, width (-)=i16 6, precision (6)=i16 2) -> (F-format string=w1383:string)  [unwired: 1 in]
            }
          }
        }
        n619 = Replace Array Subset(array=w1347, new element #1=w1341, index (col) #1=5 ("disabled index (col)"), new element #2=w1340, index (col) #2=6 ("disabled index (col)")) -> (w1345:string[][])  [unwired: 2 in]
        n620 = local write "Sub-Cycle Pattern"(w1345) -> ()
      }
      frame "Total time calc" {
        w1402 = i16 2 ("width (-)")
        w1409 = ":"
        n621 = local read "Cycle Pattern"() -> (w1416:string[][])
        n622 = Index Array(array=w1416, index (col)=4 ("disabled index (col)")) -> (element=w1389:string[])  [unwired: 1 in]
        n623 = Array Size(array=w1389) -> (size(s)=w1391:i32)
        n624 = Search 1D Array(1D array=w1389, element="") -> (index of element=w1390:i32)  [unwired: 1 in]
        n625 = Equal?(x=w1390, y=-1) -> (x = y?=w1392:bool)
        n626 = Select(t=w1391, s=w1392, f=w1390) -> (s? t:f=w1388:i32)
        n627 = for {
          N: w1388 -> [_]
          tunnel: w1389 -> [w1424] mode=indexing
          shift-right: [w1426] -> w1412
          shift-left: 0 -> [w1427]
          n628 = xnode "Match Regular Expression"("input string"=w1424, "regular expression"=":" ("search string/char (-)")) -> ("before match"=w1423:string, "after match"=w1420:string)  [unwired: 4 in, 3 out]
          n629 = Decimal String To Number(string=w1423) -> (number=w1422:i32)  [unwired: 2 in, 1 out]
          n630 = Decimal String To Number(string=w1420) -> (number=w1419:i32)  [unwired: 2 in, 1 out]
          n631 = Multiply(x=w1422, y=60) -> (x*y=w1418:i32)
          n632 = Add(x=w1418, y=w1419) -> (x+y=w1417:i32)
          n633 = Add(x=w1417, y=w1427) -> (x+y=w1426:i32)
        }
        n634 = local read "Total Number of Cycles"() -> (w1413:T1)
        n635 = Multiply(x=w1412, y=w1413) -> (x*y=w1408:T1)
        n636 = Quotient & Remainder(x=w1408, y=3600.0) -> (x-y*floor(x/y)=w1395:T1, floor(x/y)=w1405:T1)
        n637 = Quotient & Remainder(x=w1395, y=60.0) -> (x-y*floor(x/y)=w1403:T1, floor(x/y)=w1404:T1)
        n638 = Number To Decimal String(number=w1405) -> (decimal integer string=w1410:string)  [unwired: 1 in]
        n639 = Number To Decimal String(number=w1404, width (-)=w1402) -> (decimal integer string=w1406:string)
        n640 = Number To Decimal String(number=w1403, width (-)=w1402) -> (decimal integer string=w1401:string)
        n641 = Concatenate Strings(w1410, w1409, w1406, w1409, w1401) -> (w1400:string)
        n642 = call <vilib>:"Search and Replace Pattern.vi"("string"=w1400, "regular expression (\"\")"=" " ("replace string (\"\")"), "replace string (\"\")"="0" ("replace string (\"\")"), "replace all? (F)"=TRUE) -> ("result string"=→"Total Test Duration (hrs)":string)  [unwired: 1 in, 1 out]
      }
      frame "update Cycle pattern " {
        n643 = local read "Cycle Pattern"() -> (w1555:string[][])
        n644 = Index Array(array=w1555, index (col)=1 ("disabled index (col)")) -> (element=w1540:string[])  [unwired: 1 in]
        n645 = String To Path(string=w1557) -> (path=w1558:path)
        n646 = Array Size(array=w1540) -> (size(s)=w1543:i32)
        n647 = Search 1D Array(1D array=w1540, element="") -> (index of element=w1542:i32)  [unwired: 1 in]
        n648 = List Folder(path=w1558, pattern="*.eyes") -> (filenames=w1556:string[])  [unwired: 2 in, 3 out]
        n649 = Equal?(x=w1542, y=-1) -> (x = y?=w1544:bool)
        n650 = Select(t=w1543, s=w1544, f=w1542) -> (s? t:f=w1541:i32)
        n651 = for {
          N: w1541 -> [_]
          tunnel: w1555 -> [w1574] mode=indexing
          tunnel: w1557 -> [w1567]
          tunnel: [w1569] -> w1550 mode=indexing
          tunnel: [w1571] -> w1554 mode=indexing
          tunnel: [w1568] -> w1551 mode=indexing
          tunnel: w1556 -> [w1566]
          tunnel: [w1561] -> w1547 mode=indexing
          n652 = Index Array(array=w1574, index #1=1 ("index"), index #2=3 ("index")) -> (element #1=w1565:string, element #2=w1570:string)
          n653 = Search 1D Array(1D array=w1566, element=w1565) -> (index of element=w1564:i32)  [unwired: 1 in]
          n654 = Not Equal?(x=w1564, y=-1) -> (x != y?=w1562:bool)
          n655 = case shown="True" w1562 {
            tunnel: [w1578 w1592] -> w1571
            tunnel: w1570 -> [_ w1588]
            tunnel: [w1578 w1586] -> w1569
            tunnel: [w1578 w1585] -> w1568
            tunnel: w1567 -> [_ w1584]
            tunnel: w1565 -> [w1577 w1583]
            tunnel: [w1576 w1583] -> w1561
            frame False {
              w1578 = "N/A" ("String")
              n656 = Concatenate Strings(w1577, " - File NOT AVAILABLE !!!" ("string")) -> (w1576:string)
            }
            frame True {
              w1596 = i16 2 ("width (-)")
              n657 = Concatenate Strings(w1584, w1583) -> (w1614:string)
              n658 = String To Path(string=w1614) -> (path=w1613:path)
              n659 = call <vilib>:"Search and Replace Pattern.vi"("string"=w1588, "regular expression (\"\")"="[a-x ]" ("format string"), "replace string (\"\")"="", "replace all? (F)"=TRUE) -> ("result string"=w1585:string)  [unwired: 1 in, 1 out]
              n660 = call-poly <vilib>:"Read From Spreadsheet File.vi"("file path (dialog if empty)"=w1613) -> ("first row"=w1582:string[])  [unwired: 6 in, 4 out]
              n661 = Delete From Array(array=w1582, length=1, index=0) -> (array with subset deleted=w1581:string[])  [unwired: 1 out]
              n662 = Array Size(array=w1581) -> (size(s)=w1612:i32)
              n663 = Equal?(x=w1585, y="") -> (x = y?=w1600:bool)
              n664 = Subtract(x=w1612, y=12) -> (x-y=w1610:i32)
              n665 = Select(t="0", s=w1600, f=w1585) -> (s? t:f=w1599:string)
              n666 = Index Array(array=w1581, index=w1610) -> (element=w1586:string)
              n667 = Decimal String To Number(string=w1599) -> (number=w1609:i32)  [unwired: 2 in, 1 out]
              n668 = Decimal String To Number(string=w1586) -> (number=w1608:i32)  [unwired: 2 in, 1 out]
              n669 = Multiply(x=w1609, y=w1608) -> (x*y=w1607:i32)
              n670 = Quotient & Remainder(x=w1607, y=60) -> (x-y*floor(x/y)=w1605:i32, floor(x/y)=w1604:i32)
              n671 = Number To Decimal String(number=w1605, width (-)=w1596) -> (decimal integer string=w1602:string)
              n672 = Number To Decimal String(number=w1604, width (-)=w1596) -> (decimal integer string=w1601:string)
              n673 = Concatenate Strings(w1601, ":", w1602) -> (w1595:string)
              n674 = call <vilib>:"Search and Replace Pattern.vi"("string"=w1595, "regular expression (\"\")"=" " ("replace string (\"\")"), "replace string (\"\")"="0" ("replace string (\"\")"), "replace all? (F)"=TRUE) -> ("result string"=w1592:string)  [unwired: 1 in, 1 out]
            }
          }
        }
        n675 = Replace Array Subset(array=w1555, new element #1=w1547, index (col) #1=1 ("disabled index (col)"), new element #2=w1550, index (col) #2=2 ("disabled index (col)"), new element #3=w1551, index (col) #3=3 ("disabled index (col)"), new element #4=w1554, index (col) #4=4 ("disabled index (col)")) -> (w1559:string[][])  [unwired: 4 in]
        n676 = local write "Cycle Pattern"(w1559) -> ()
      }
      frame "load cycle name" {
        n677 = property on="Cycle Pattern" class="Tbl (strict)"() -> ("EditPos"=w1620:T3)  [unwired: 2 in, 2 out]
        n678 = Unbundle By Name(w1620) -> ("Row"=w1618:i32, "Column"=w1617:i32)
        n679 = local read "Cycle Pattern"() -> (w1616:string[][])
        n680 = call "SubCycles list.vi"() -> ("Subcycle name"=w1619:string)  [unwired: 10 in, 1 out]
        n681 = Replace Array Subset(array=w1616, new element=w1619, index (row)=w1618, index (col)=w1617) -> (w1615:string[][])
        n682 = local write "Cycle Pattern"(w1615) -> ()
      }
      frame "load test array" {
        n683 = local read "Total Test Duration (hrs)"() -> (w1628:T8)
        n684 = local read "Cycle Name"() -> (w1624:T5)
        n685 = Equal?(x=w1624, y="") -> (x = y?=w1623:bool)
        n686 = Not Equal?(x=w1628, y="0:00:00") -> (x != y?=w1622:bool)
        n687 = Or(x=w1622, y=w1623) -> (x .or. y?=w1621:bool)
        n688 = case shown="True" w1621 {
          selector: w1621 -> [w1629 _]
          tunnel: [FALSE TRUE] -> w1626
          frame False {
            n689 = case shown="False" w1629 {
              frame False {
                n690 = One Button Dialog(message="Incomplete Data!\nReview the cycle pattern!") -> ()  [unwired: 1 in, 1 out]
              }
              frame True {
              }
            }
          }
          frame True {
            w1635 = 0.0 ("default (0 I32)")
            n691 = local read "Cycle Name"() -> (w1650:T5)
            n692 = Concatenate Strings("C:\\Setup Files\\Cycles Folder\\", w1650, ".eyec" ("string")) -> (w1648:string)
            n693 = String To Path(string=w1648) -> (path=w1649:path)
            n694 = local read "Total Number of Cycles"() -> (w1646:T1)
            n695 = call-poly <vilib>:"Read From Spreadsheet File.vi"("file path (dialog if empty)"=w1649) -> ("first row"=w1632:string[])  [unwired: 6 in, 4 out]
            n696 = call "Remove names.vi"("Array in"=w1632) -> ("Array out"=w1641:string[])  [unwired: 10 in]
            n697 = Index Array(array=w1632, index #1=14 ("index"), index #2=15 ("index")) -> (element #1=w1637:string, element #2=w1633:string)
            n698 = Number To Decimal String(number="Ageing Gas") -> (decimal integer string=w1645:string)  [unwired: 1 in]
            n699 = Number To Decimal String(number=w1646) -> (decimal integer string=w1644:string)  [unwired: 1 in]
            n700 = Decimal String To Number(string=w1633, default (0L)=w1635) -> (number=w1634:dbl)  [unwired: 1 in, 1 out]
            n701 = Decimal String To Number(string=w1637, default (0L)=w1635) -> (number=w1636:dbl)  [unwired: 1 in, 1 out]
            n702 = property on="Inlet temp Age" class="DigNum (strict)"("Value"=w1636) -> ()  [unwired: 2 in, 2 out]
            n703 = property on="Flow rate Age" class="DigNum (strict)"("Value"=w1634) -> ()  [unwired: 2 in, 2 out]
            n704 = Build Array (concatenate)(w1645, w1644, w1641) -> (w1640:string[])
            n705 = shared-variable "RT CompactRIO Target 2\\Library 1.lvlib\\Ageing Variables"(w1640) -> ()  [unwired: 1 in, 1 out]
          }
        }
        "Test Compiled" <- w1626
      }
      frame "convert to num" {
        n706 = local read "EditPos Subc"() -> (w1655:T3)
        n707 = Unbundle By Name(w1655) -> ("Row"=w1656:i32, "Column"=w1653:i32)
        n708 = Equal?(x=w1653, y=7) -> (x = y?=w1652:bool)
        n709 = case shown="False" w1652 {
          tunnel: w1656 -> [_ w1661]
          tunnel: w1653 -> [_ w1659]
          tunnel: w1655 -> [_ _]
          frame True {
          }
          frame False {
            n710 = local read "Sub-Cycle Pattern"() -> (w1658:string[][])
            n711 = call "Conv to num.vi"("Column"=w1659, "Row"=w1661, "Array"=w1658) -> ("result string"=w1660:string)  [unwired: 8 in]
            n712 = Replace Array Subset(array=w1658, new element=w1660, index (row)=w1661, index (col)=w1659) -> (w1657:string[][])
            n713 = local write "Sub-Cycle Pattern"(w1657) -> ()
          }
        }
      }
      frame "check scycle name" {
        n714 = local read "Sub-Cycle Name"() -> (w1662:T5)
        n715 = call <vilib>:"Search and Replace Pattern.vi"("string"=w1662, "regular expression (\"\")"="[^0-9a-zA-Z ]" ("format string"), "replace string (\"\")"="", "replace all? (F)"=TRUE) -> ("result string"=w1668:string)  [unwired: 1 in, 1 out]
        n716 = Not Equal?(x=w1668, y=w1662) -> (x != y?=w1667:bool)
        n717 = case shown="False" w1667 {
          tunnel: w1668 -> [w1669 w1670]
          tunnel: [w1669 w1670] -> w1663
          frame False {
          }
          frame True {
            n718 = One Button Dialog(message="Unsuitable character for the file name!") -> ()  [unwired: 1 in, 1 out]
          }
        }
        n719 = local write "Sub-Cycle Name"(w1663) -> ()
      }
      frame "check cycle name" {
        n720 = local read "Cycle Name"() -> (w1672:T5)
        n721 = call <vilib>:"Search and Replace Pattern.vi"("string"=w1672, "regular expression (\"\")"="[^0-9a-zA-Z ]" ("format string"), "replace string (\"\")"="", "replace all? (F)"=TRUE) -> ("result string"=w1678:string)  [unwired: 1 in, 1 out]
        n722 = Not Equal?(x=w1678, y=w1672) -> (x != y?=w1677:bool)
        n723 = case shown="False" w1677 {
          tunnel: w1678 -> [w1679 w1680]
          tunnel: [w1679 w1680] -> w1673
          frame False {
          }
          frame True {
            n724 = One Button Dialog(message="Unsuitable character for the file name!") -> ()  [unwired: 1 in, 1 out]
          }
        }
        n725 = local write "Cycle Name"(w1673) -> ()
      }
      frame "Multigas connect" {
        # "add here logic to verify the user requirements and the machine state\n0 - not connected\n1 - MKS1 & Ext An Up\n2 - MKS2 & Ext An Dn\n3 - MKS 1 & 2  & Ext An Up & Dn"
        n726 = flat-sequence {
          frame #0 {
            "Connected?" <- TRUE
          }
        }
      }
      frame "Multigas disconnect" {
      }
      frame "Leak Test" {
        n727 = call "Press_Test.vi"() -> ("Reset Button"=w1683:bool)  [unwired: 11 in]
        n728 = local write "Leak Test"(w1683) -> ()
      }
    }
    n729 = local read "stop 2"() -> (w1058:bool)
  }
  n730 = node-c288(w7) -> ()  [unwired: 1 out]
  n731 = local write "stop 2"(w16) -> ()
  n732 = node-c288(w14) -> ()  [unwired: 1 out]
  "Table" <- string[][] [] ("Table")
